vi "SetList.vi"() -> ()   [LabVIEW 2013]
uses:
  ColumnVIs/Column/Column.lvclass
  ColumnVIs/ModeCol/ModeCol.lvclass
  ColumnVIs/GroupCol/GroupCol.lvclass
  ColumnVIs/DigitalCol/DigitalCol.lvclass
  ColumnVIs/TriggerCol/TriggerCol.lvclass
  ColumnVIs/SingleValCol/SingleValCol.lvclass
  <vilib>/event_ctls.llb/eventvkey.ctl
  <vilib>/Utility/miscctls.llb/LVRowAndColumnTypeDef.ctl
  TypeDefs/RowType.ctl
  TypeDefs/TableHistory.ctl
  TypeDefs/TableArray.ctl
  TypeDefs/AddDeviceRing.ctl
  DeviceVIs/Device/Device.lvclass
  TypeDefs/PreviousVersionSelect.ctl
  VariableManagerCodes/VariableManager/VariableManager.lvclass
  <vilib>/Utility/miscctls.llb/LVRowAndColumnUnsignedTypeDef.ctl
  PackedLibraries/LuaEvaluatorAPI.lvlibp/API/t_Caching_Expression_Evaluator_Methods_Table.ctl
  TypeDefs/ClickEvent.ctl
  <vilib>/Utility/miscctls.llb/LVPoint32TypeDef.ctl
  TypeDefs/SetListRefs.ctl
  <vilib>/Utility/error.llb/DialogType.ctl
  TypeDefs/SaveCluster.ctl
  <vilib>/Utility/miscctls.llb/LVStringsAndValuesArrayTypeDef_I32.ctl
  <vilib>/Utility/cursorutil.llb/Set Cursor (Icon Pict).vi
  VariableManagerCodes/API/VariableManagerAPI.lvlib
  Globals/UserFunctions.vi
  PackedLibraries/LuaEvaluatorAPI.lvlibp
panel:
  in  "Launch Viewer":bool
  out "Cycle Time (s)":dbl
  in  "UpdateHWI Button":bool
  in  "StopExperiment":bool
  in  "Run Seq Button":bool
  in  "Run Button":bool
  in  "Cycle":bool
  in  "RandomSequence":bool
  out "Procedure Name":string="test_branch"
  in  "Tab Control":T1(tab)=enum."Variables"
  in  "Resume Button":bool
  in  "Program only changes":bool=TRUE
  out "SequenceHistory":string[][](table)
  in  "File Number":i32
  in  "Program during MOT loading":bool
  in  "Additional wait time (s)":dbl
  out "Igor Inform String":string
  in  "FitCol2Text Button":bool
  in  "SetList Table":string[][](table)=[["initialize", "", "Ramp", "1", "1", "0", "0", "0", "0", "0", "0", "0", "0", "0", "0", "0", "0", "0", "0", "0", "0", "0", "0", "0", "0", "0", "0", "0", "0", "100m"]]
  in  "Undo":bool
  in  "Redo":bool
  in  "Select Layout":i32(ring)=-1 items=["(On-the-fly)"=-2, "All"=-1]
  in  "ConfigLayoutsButton":bool
  in  "Add Device":T2 items=["Select Type...", "DDS", "Novatech", "NI Card", "Slave PB", "PTS via PB"]
  in  "ManageDevicesButton":bool
  in  "User defined functions":string="-- --------------------------------------------------------------------------\n-- RbYb Beatnote Command \"frequency\" functions\n--      These functions allow us to run a sequence using absolute frequency \n--      detuning by calculating the proper command \"frequency\"\n--\n--      NOTE: Only use one TA or Re \"comm\" function, or it isn't clear which setpoint will be used\n--\n--      18.Aug.2010: Updated Master AOM offset (40 --> 42.342).\n-----------------------------------------------------------------------------\nfunction TASlowComm(Detuning,AOM)\n    return (-1*Detuning+1126.48-60.32-42.342-2*AOM)/8\n   --positive detuning is BLUE detuned, zero detuning sets TA slower beam to the 87-Rb F=2 to F'=3\nend\n\nfunction TAMOTComm(Detuning,AOM)\n    return (-1*Detuning+1126.48-60.32-42.342+AOM)/8\n   --positive detuning is BLUE detuned, zero detuning sets TA MOT beam to the 87-Rb F=2 to F'=3\nend\n\nfunction TAPComm(Detuning,AOM)\n    return (-1*Detuning+1126.48-60.32-42.342+AOM)/8\n   --positive detuning is BLUE detuned, zero detuning sets TA Probe beam to the 87-Rb F=2 to F'=3\nend\n\nfunction ReMOTComm(Detuning,AOM)\n    return (Detuning+6568.03-1126.48+60.32+42.342-2*AOM)/64\n    --positive detuning is BLUE detuned, zero detuning sets Repump MOT beam to the 87-Rb F=1 to F'=2\nend\n\nfunction ReSlowComm(Detuning,AOM)\n    return (Detuning+6568.03-1126.48+60.32+42.342+2*AOM)/64\n    --positive detuning is BLUE detuned, zero detuning sets Repump slower beam to the 87-Rb F=1 to F'=2\nend\n\n--RbLi Probe (transverse coolign launch)\nfunction PComm(Detuning)\n    return (-1*Detuning+986.16)/8\n    --positive detuning is BLUE detuned, zero detuning sets Repump slower beam to the 87-Rb F=1 to F'=2\nend\n\n-- Creates an exponential ramp from A to B in tEnd seconds\n-- useful for stopping a ramp at different times to measure T, N\nfunction ExpRampStep(t, a, b, tau, tEnd)\n   return (b - a*exp(tEnd / tau) + (a-b)*exp(t/tau))/ ( 1 - exp(tEnd / tau) );\nend\n\nfunction ExpRampEnd(tEv, a, b, tau, tEnd)\n   return (b - a*exp(tEnd / tau) + (a-b)*exp(tEv/tau))/ ( 1 - exp(tEnd / tau) );\nend\n\nfunction ExpRamp2(t,a,tau)\n   return a*exp(-t/tau)\nend\n\nfunction ExpRamp2End(tEnd,a,tau)\n   return a*exp(-tEnd/tau)\nend\n\n-- Added log chip amplifier (1 V per decade) so now we provide linear ramp to get exponential\n--     note: log() is base 'e', log10 base '10'\nfunction LineEvap(t,a,tau)\n   return 1.027*(log10(a)-t/(2.30*tau))+0.0343\nend\n\n-- final value log(V) for LineEvap\nfunction LineEvapEnd(tEnd,a,tau)\n   return 1.027*(log10(a)-tEnd/(2.30*tau))+0.0343\nend\n\n-- Convert real dipole power to log chip request V\nfunction PtoV(pow)\n   return 1.010*log10(pow/0.770)\nend\n\n-- Convert 532 horizontal (main) beam power (in mW) to V-req\nfunction PtoV532m(pow)\n   return 1.01378*log10(pow/0.54672)\nend\n\n-- Convert 532 vertical (crossing) beam power (in mW) to V-req\nfunction PtoV532c(pow)\n   return 1.03459*log10(pow/0.619665)\nend\n\n-- Convert 1064 horizontal (main) beam power (in mW) to V-req\nfunction PtoV1064m(pow)\n   return 1.0035*log10(pow/1.2104)\nend\n----------------------------------------\n-- The following functions are part of the \"standard load\" of functions and should not be messed with\n-- They are here for reference only.\n-- Please add any user functions above this comment\n-- -------------------------------------------------------------------------------------------\n\n-- Creates a linear ramp from A to B\nfunction LineRamp(f, Initial, Final)\n    return (1-f)*Initial + f*Final;\nend\n\n-- Creates an exponential ramp from A to B\nfunction ExpRamp(t, a, b, tau)\n   return (b - a*exp(tMax / tau) + (a-b)*exp(t/tau))/ ( 1 - exp(tMax / tau) );\nend\n\n-- Creates a sinewave\nfunction SinRamp(t,Offset,A,Freq, Phase)\n    return Offset + A * sin(2*pi*Freq*t + Phase)\nend\n\n-- Creates a blackman pulse\nfunction Blackman(f, Offset, A)\n    return Offset +  A*sqrt(0.5*cos(3.1415*(2*f-1))+0.08*cos(2*pi*(2*f-1))+0.42);\nend\n\n-- Creates a half-gauss ramp\nfunction HalfGaussRamp(t, a, b, Width)\n    local y;\n    y = exp(-(tMax^2)/Width^2);\n    y = (a -  b*y)/(1-y)  +  ((b-a)/(1-y))*exp(-((t-tMax)^2)/Width^2);\n    return y;\nend\n\n-- Creates an \"O'Hara\" ramp from A to B, for dipole evaporation\nfunction EvapRamp(t, a, b, tau)\n   local y;\n  y = log(a/b) / log(1+tMax/tau);\n  y = a * (1+t/tau)^(-y);\n  return y;\nend\n"
  out "Loading Text":string="Loading..."
  in  "Version Selection":T3=enum."Load DDS 4.10"
  in  "Old HWGlobals Path":path=path "C:/Experiment/Data Acquisition/Hardware Control/Hardware/2014/6Jun2014_PowerCal" caption="This file has not been loaded or saved"
  in  "Old HWGlobals History":string(combo)
  in  "Old Procedure Path":path=path "C:/Experiment/Data Acquisition/Hardware Control/procedures/Benchmarks/12Feb2014_RbQuad" caption="This file has not been loaded or saved"
  in  "Old Procedure History":string(combo)
  in  "Load Old":bool
  in  "Load Recent":string(combo)
  in  "Save to Disk":bool
  in  "Load from Disk":bool
  out "Loaded Version":string="testing"
  out "Table error":errorcluster
  out "Run/Sequence Error":errorcluster
  out "Update Error":errorcluster
  out "Index Values":T4
  out "#chg":i16
  out "Defer Pnl Upd":bool=TRUE
  out "diag. loop cnt":i32
  out "Key Focus":bool
  out "Edit Position":T5={"Row"=-2, "Column"=-2}
  out "withinSelection?":bool
  out "Val Change":bool=TRUE
  out "Selection Size":T5
  out "Selection Start":T5={"Row"=25, "Column"=30}
  out "Char":i16
  out "VKey":T6
  out "withinData?":bool=TRUE
  out "data cols":i32=134
  out "data rows":i32=26
  out "Number of Rows":u32=36
  out "Number of Columns":u32=62
  in  "Devices":refnum<class "Device.lvclass">[](array[class])
  out "Devices queue":refnum<queue>
  out "DevNums":i32[](array[numeric])=[0, 0, 0, 0, 0, 0, 0, 0, 0, 0, 0, 0, 0, 0, 0, 0, 0, 0, 0, 0, 0, 0, 0, 0, 0, 0, 0, 0, 0, 0, 1, 1, 1, 1, 1, 1, 1, 1, 1, 1, 1, 1, 1, 1, 1, 1, 1, 1, 1, 1, 2, 2, 2, 2, 2, 2, 2, 2, 2, 2, 2, 2, 2, 2, 2, 2, 2, 2, 2, 2, 3, 3, 3, 3, 3, 3, 3, 3, 3, 3, 3, 3, 3, 3, 3, 3, 3, 3, 3, 3, 4, 4, 4, 4, 4, 4, 4, 4, 5, 5, 5, 5, 5, 5, 5, 5, 5, 5, 5, 5, 6, 6, 6, 6, 6, 6, 6, 6, 6, 6, 6, 6, 7, 7, 7, 7, 7, 7, 7, 7, 7, 7, 7, 7]
  out "Col array":refnum<class "Column.lvclass">[](array[class])
  out "Seq. Event":refnum<user-event>
  out "Update Event":refnum<user-event>
  out "Update Notifier":refnum<notifier>
  out "Dyn. Regist. Update Event":refnum<event-registration>
  out "Dyn.\nRegist.\nSeq.\nEvent":refnum<event-registration>
  out "Dyn.\nRegist.\nCycleX\nEvent":refnum<event-registration>
  out "CycleX Event":refnum<user-event>
  in  "row type":T7=enum."within data"
  out "Button\n(Mouse Down?)":u16
  in  "VariableManager":refnum<class "VariableManager.lvclass">=refnum
  out "Igor Inform Array":string[](array[string])
  out "Clipboard":string[][](array[string])
  out "Table History":T8
  in  "Diag. loop?":bool
  in  "PreserveHist?":bool
  out "Hist. size":i32=2
  in  "Defer Updates?":bool=TRUE
  in  "initialize?":bool
  in  "Debug: apply appearance":bool
  out "Viewer VI ref":refnum<vi>
  in  "quit":bool
  # "What do we actually need from old CycleX here?\n   - Inform Igor?\n   - Program changes/ during MOT load?"
  # "(not presently implemented)"
  # "Variable Manager will be initialized when the VI is run.\n\nIf it is currently running and you can see this message, then you've \"popped out\" the Variable manager.\nClose it with the \"red-x\" to replace it here."
  # "Note: For each index <idx>, the names <idx>_f and <idx>_max\nare also defined as the fractional sequence step and max steps."
  # "NOTE: these persist until LabVIEW is closed or you overwrite them."
  # "In the context of ramps several variables are passed or specified that may be used here:\n\n   - f the fractional position of a point in a ramp\n   - t the current time in a ramp\n   - dt the current timestep size.\n   - tMax the total duration of the ramp\n\ntemporary \"storage\":\n-- not functionality for strings (always treated as double)\nfunction bnot(a)\n   -- this \"(bool exp.) and b or c\" is equivalent to \"(bool exp.) ? b : c\" syntax.\n   -- caution: undefined variables evaluate to \"false\" so will NOT throw an error as argument\n   return a==0 and 1 or 0\nend"
  # "Present Version"
  # "Save/Load from present version (select single file):\nWe need to save the following:\n   - Devices (with the columns and data pushed from table first!)\n   - Layout ring (for layout names, #s)\n   - variables\n   - user functions\n   - ... ?"
  # "Load... and Save... bring up dialog box.\nLoad Recent will load the selected procedure. BUG: not a value change if select what's on top!"
  # "Previous Versions"
  # "Load from older versions (select Procedure and Hardware globals)\n(1) reformat old file to give device array\n(2) collect variables and send them to variable manager\n(3) load user functions\n(4) construct layouts, if any (at least a default \"all on\" layout)\n(5) ...?"
  # "Most of these controls/indicators MUST exist. At the bottom and right are some diagnostics."
  # "\"Diagnostics\" we can't delete:\nRow Type, ..."
  # "(must abort to stop,\nstill better to QUIT first)"
  # "diagnostics:"
  # "presently not set\nfor row header"
  # "The table size in (rows, cols) is NOT same as\nthe size of the data array displayed in table."
  # "SetList was developed for the JQI neutral atom cooling/traping groups. \nPrimary contributions authored by Zack Seigel, Creston Herold, Joe Tiamsuphat, Bob Wyllie, Zach Smith.\n\nFAQs\n------\n * How are digital variables interpreted?\n     Any value not equal to 0 is high, only 0 is low.\n\n * What does Ramp mean?\n     Slave devices will be triggered (if necessary) during a Ramp line with a period given by \"Step.\" The output\n     is determined with Lua \"User Functions\" and the reserved f,t variables described on that tab.\n     Master (PulseBlaster) channels will output a *static* output during ramps. That means functions of f or t\n     will only be evaluated at their *first* point for Master channels.\n\n * How do you use Loop - EndLoop?\n     The \"Step\" column on a Loop line is for # loops and is ignored on an EndLoop line. Nesting is supported\n     up to 7 levels deep, but only Master (PulseBlaster) outputs can change. Therefore Ramps are not allowed \n     within loops.\n\n * How does Halt work?\n     On a Halt line, the Master (PulseBlaster) will change to the selected outputs and then wait for a trigger.\n     Upon receiving a trigger (hardware or software), it will wait for the specified Delay and then go to the \n     next instruction.\n\n * Where can I learn more?\n     Complete documentation of this code, including adding your own custom device can be found on the\n     JQI wiki (https://jqi-wiki.physics.umd.edu, login required)."
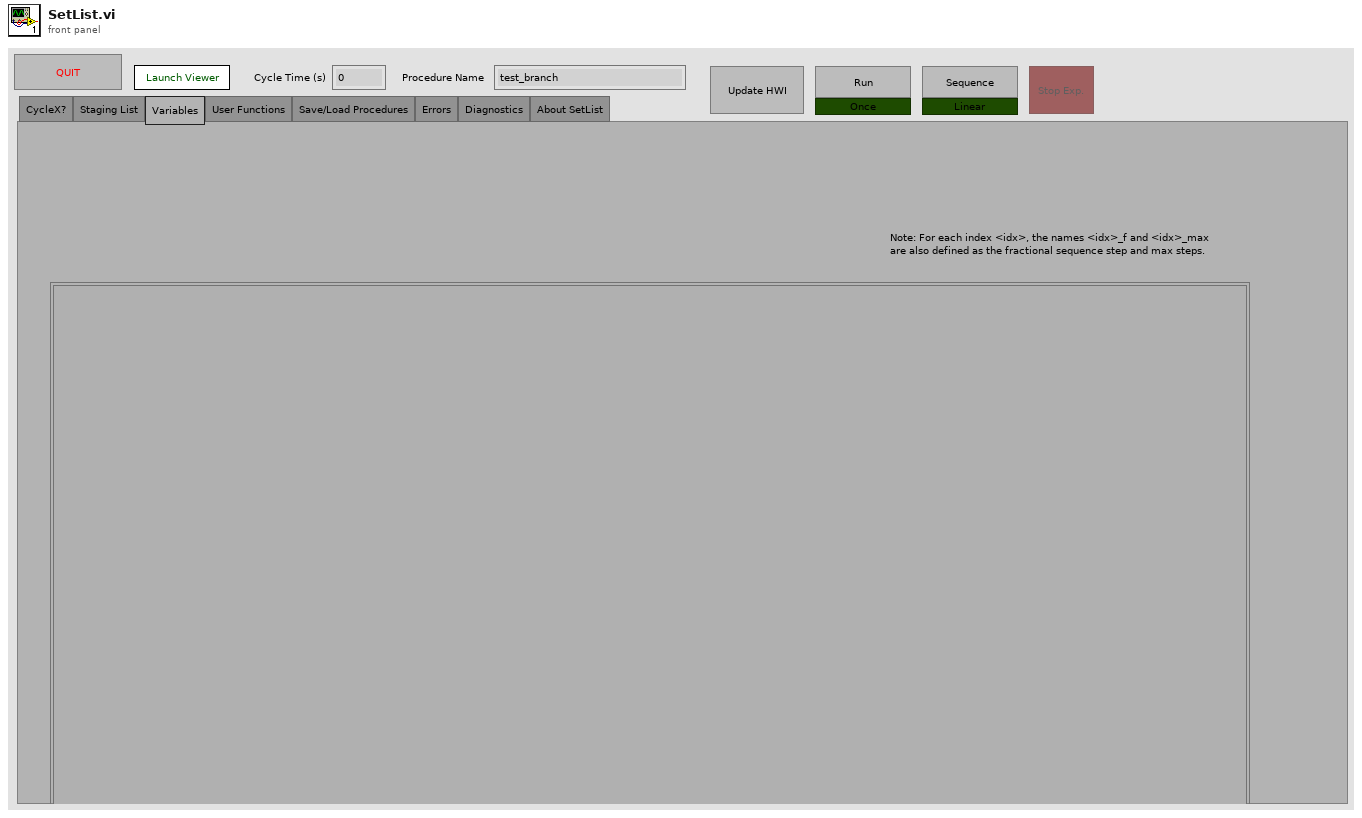
[diagram p1: front panel]
types:
  T1 = enum32{"CycleX?", "Staging List", "Variables", "User Functions", "Save/Load Procedures", "Errors", "Diagnostics", "About SetList"}
  T2 = typedef "AddDeviceRing.ctl" = u16
  T3 = typedef "PreviousVersionSelect.ctl" = enum32{"Load PreDDS 4.10", "Load early 2009 files", "Load 2009-2010 files", "Load DDS 4.10", "Load v4.09"}
  T4 = typedef "LVRowAndColumnUnsignedTypeDef.ctl" = cluster{"Row":u32, "Column":u32}
  T5 = typedef "LVRowAndColumnTypeDef.ctl" = cluster{"Row":i32, "Column":i32}
  T6 = typedef "eventvkey.ctl" = enum16{"ASCII", "Enter", "Return", "Shift", "Ctrl", "Alt", "Cmd", "Opt", "Caps", "NumLock", "Clear", "Break", "Up", "Down", "Left", "Right", "Insert", "Delete", "Home", "End", "PageUp", "PageDown", "Escape", "Help", "Pause", "ScrollLock", "F1", "F2", "F3", "F4", "F5", "F6", "F7", "F8", "F9", "F10", "F11", "F12", "F13", "F14", "F15", "F16", "F17", "F18", "F19", "F20", "F21", "F22", "F23", "F24", "Play", "VolumeUp", "VolumeDown", "Mute", "Two Byte Char"}
  T7 = typedef "RowType.ctl" = enum16{"below data", "within data", "column header", "first row"}
  T8 = typedef "TableHistory.ctl" = cluster{"OldTable Array":T9, "Undo pointer":i32}
  T9 = typedef "TableArray.ctl" = cluster{"OldTable":string[][]}[]
  T10 = typedef "LuaEvaluatorAPI.lvlibp/t_Caching_Expression_Evaluator_Methods_Table.ctl" = enum16{"set", "get", "eval", "assign", "isvalid", "execute", "evaltable", "close"}
  T11 = enum8{"Enabled", "Disabled", "Disabled and Grayed Out"}
  T12 = typedef "ClickEvent.ctl" = cluster{"CtlRef":refnum<vi>, "Coords":T13, "Button":u16, "Mods":cluster{"Double Click":bool, "Menu Key":bool}, "PlatMods":cluster{"Shift":bool, "Ctrl":bool, "Alt":bool, "Cmd":bool, "Opt":bool}}
  T13 = typedef "LVPoint32TypeDef.ctl" = cluster{"Horizontal":i32, "Vertical":i32}
  T14 = typedef "SetListRefs.ctl" = cluster{"Clipboard":refnum<vi>, "Layout Ring Refnum":refnum<vi>, "Col Array Ref in":refnum<vi>, "VariableManagerRef":refnum<vi>, "Table CtlRef In":refnum<vi>, "Table History ref":refnum<vi>, "Devices queue":refnum<queue>}
  T15 = typedef "SaveCluster.ctl" = cluster{"Version":string, "Devices":refnum<class "Device.lvclass">[], "Select Layout":i32, "Layout:Strings And Values []":T16, "User defined functions":string, "VariableManager":refnum<class "VariableManager.lvclass">}
  T16 = typedef "LVStringsAndValuesArrayTypeDef_I32.ctl" = cluster{"String":string, "Value":i32}[]
  T17 = cluster{"Shift":bool, "Ctrl":bool, "Alt":bool, "Cmd":bool, "Opt":bool}
  T18 = typedef "ClickReturn.ctl" = cluster{"Button":u16, "Mods":cluster{"Double Click":bool, "Menu Key":bool}, "PlatMods":cluster{"Shift":bool, "Ctrl":bool, "Alt":bool, "Cmd":bool, "Opt":bool}, "Discard?":bool}
  T19 = typedef "DialogType.ctl" = u16
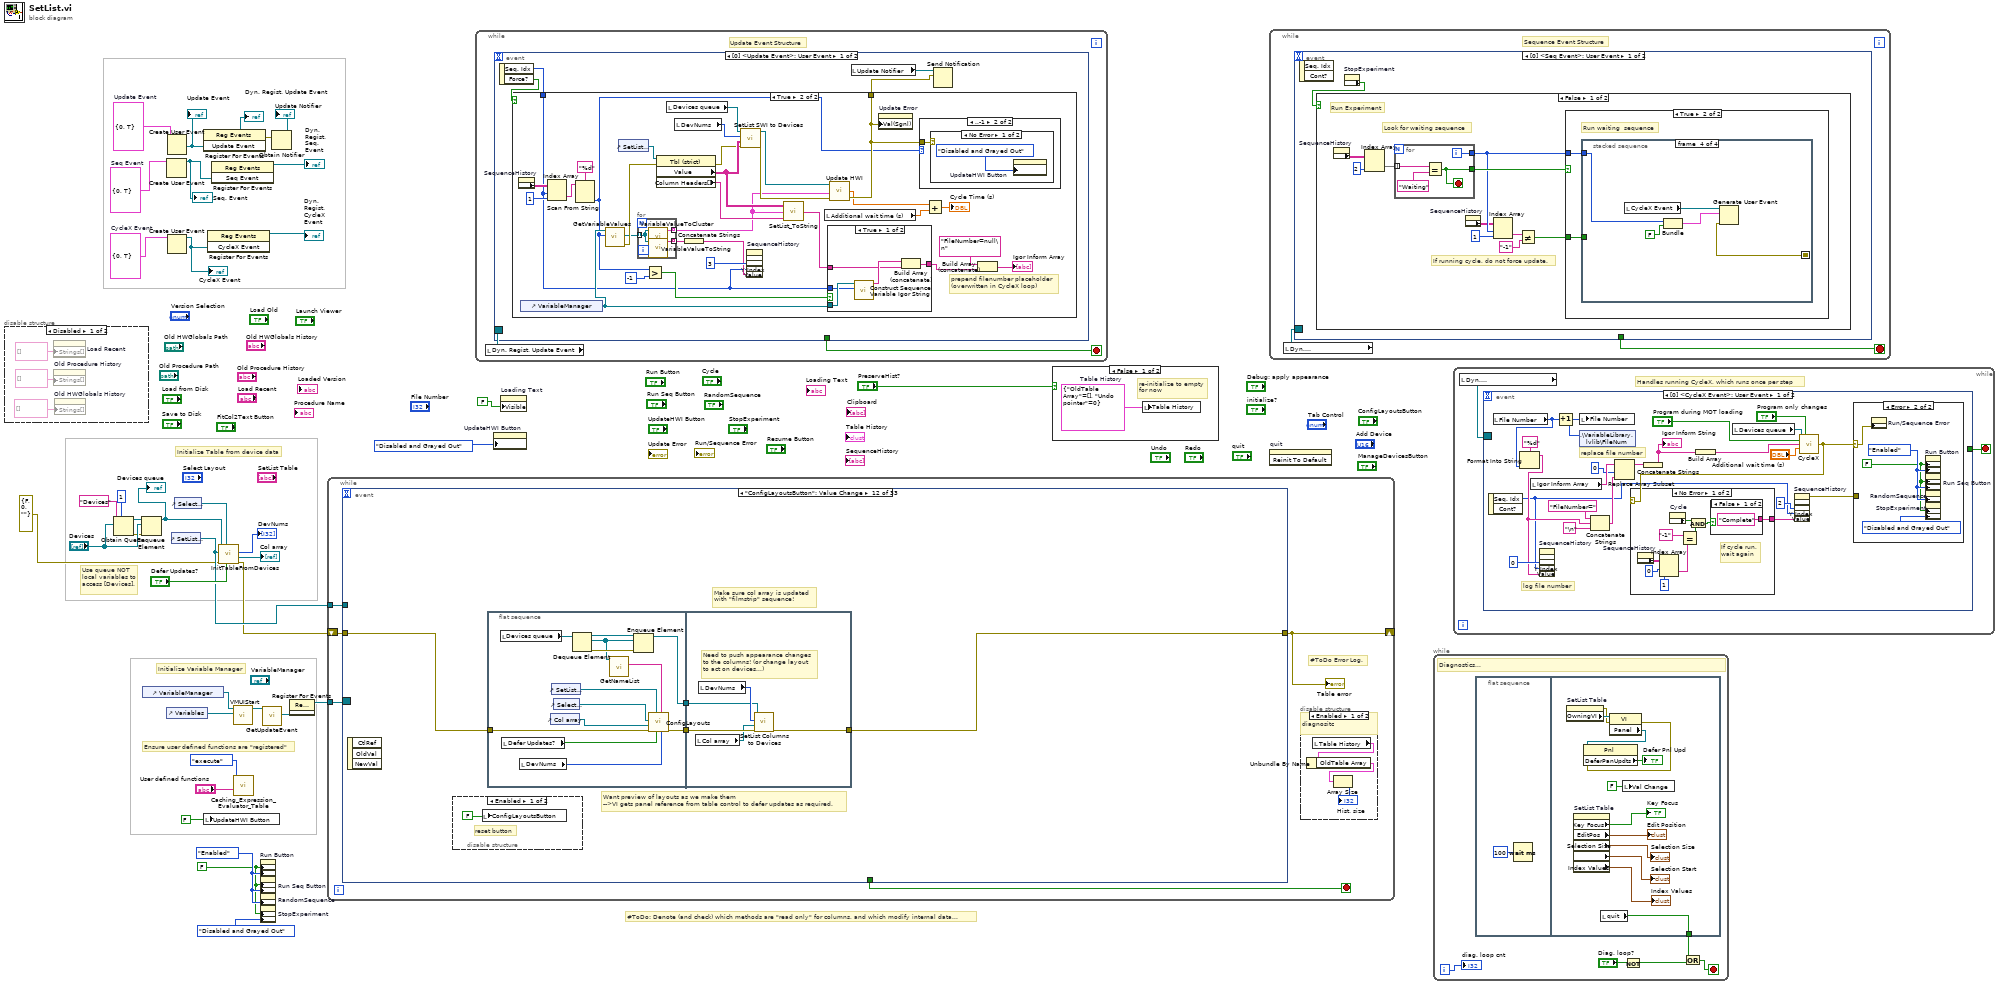
[diagram p0: block diagram]
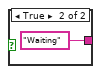
[diagram p2: hidden frame]
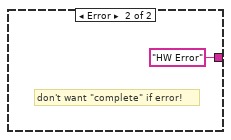
[diagram p3: hidden frame]
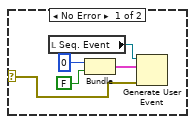
[diagram p4: hidden frame]
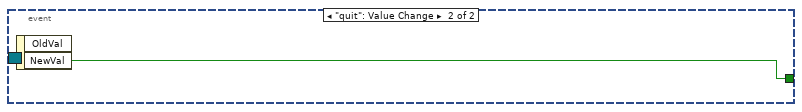
[diagram p5: hidden frame]
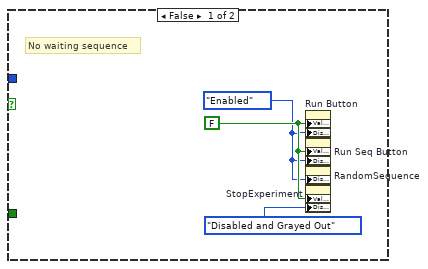
[diagram p7: hidden frame]
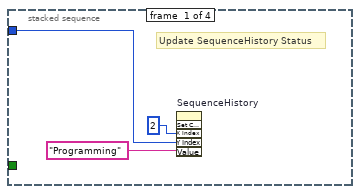
[diagram p8: hidden frame]
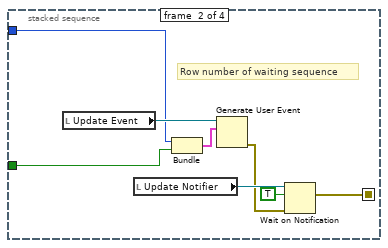
[diagram p9: hidden frame]
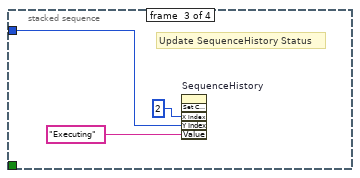
[diagram p10: hidden frame]
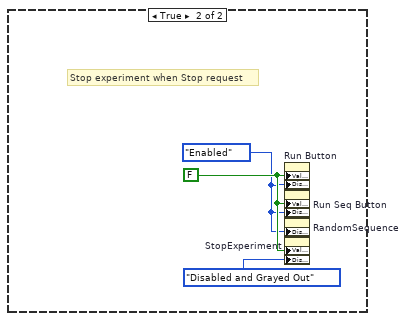
[diagram p11: hidden frame]
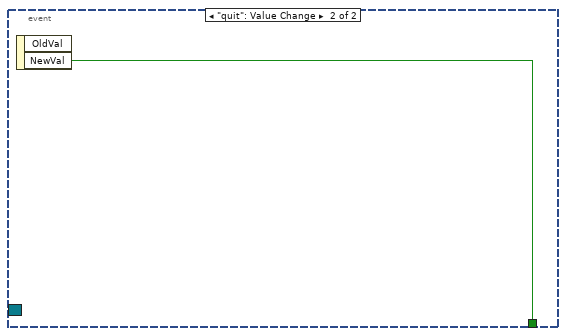
[diagram p12: hidden frame]
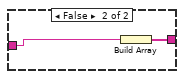
[diagram p16: hidden frame]
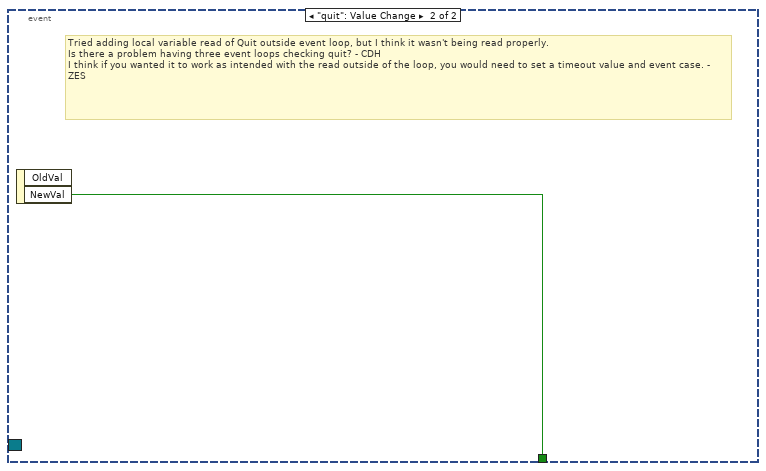
[diagram p17: hidden frame]
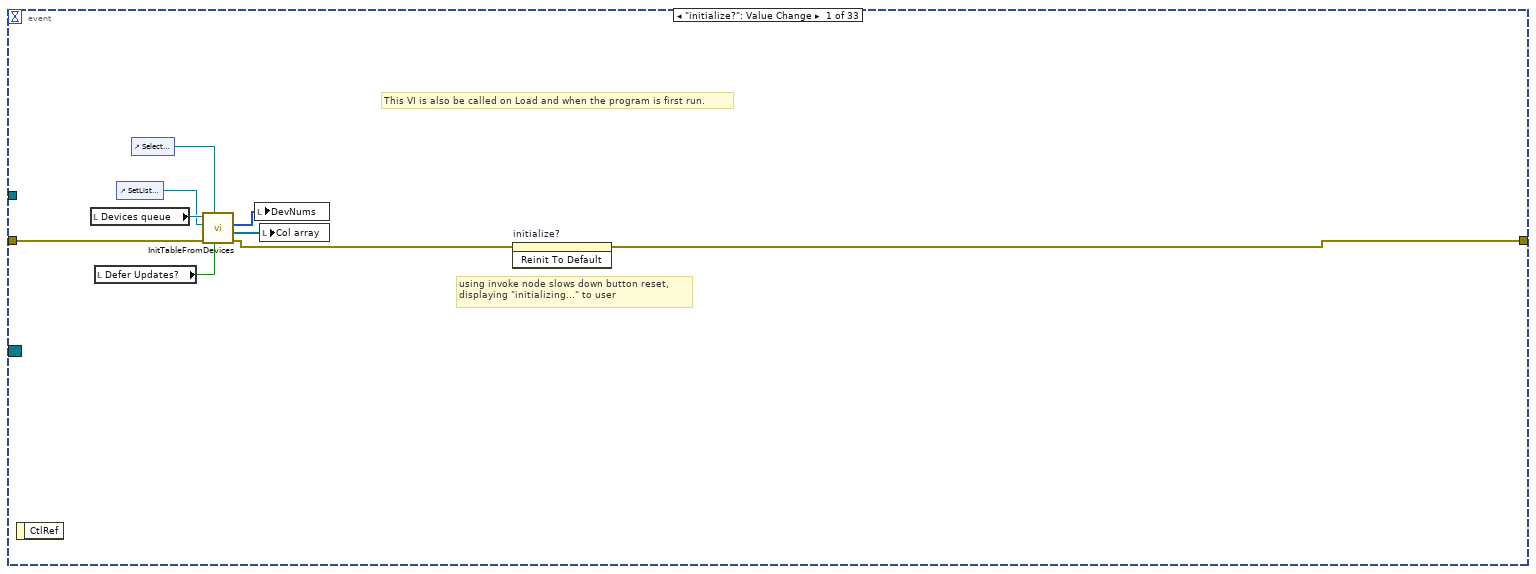
[diagram p20: hidden frame]
diagram:
  w14 = T11."Enabled" ("Disabled")
  w13 = FALSE
  w25 = cluster{"Seq. Idx":i32, "Cont?":bool} {"Seq. Idx"=0, "Cont?"=TRUE}  # CycleX Event
  w35 = cluster{"Seq. Idx":i32, "Cont?":bool} {"Seq. Idx"=0, "Cont?"=TRUE}  # Seq Event
  w36 = cluster{"Seq. Idx":i32, "Force?":bool} {"Seq. Idx"=0, "Force?"=TRUE}  # Update Event
  # "Use queue NOT\nlocal variables to\naccess [Devices]."
  # "Ensure user defined functions are \"registered\""
  # "Initialize Variable Manager"
  # "Initialize Table from device data"
  # "#ToDo: Denote (and check) which methods are \"read only\" for columns, and which modify internal data..."
  n1 = disable-structure shown="Disabled" {
    frame Disabled {
      n2 = property on="Load Recent" class="CmbBox"("Strings[]"=string[] [] ("Strings []")) -> ()  [unwired: 2 in, 2 out]
      n3 = property on="Old Procedure History" class="CmbBox"("Strings[]"=string[] [] ("Strings []")) -> ()  [unwired: 2 in, 2 out]
      n4 = property on="Old HWGlobals History" class="CmbBox"("Strings[]"=string[] [] ("Strings []")) -> ()  [unwired: 2 in, 2 out]
    }
    frame Enabled {
    }
  }
  n5 = Obtain Queue(max queue size (-1, unlimited)=1, name (unnamed)="Devices", element data type="Devices") -> (queue out=w6:refnum<queue>, error out=w5:errorcluster)  [unwired: 2 in, 1 out]
  n6 = Enqueue Element(queue=w6, element="Devices", error in (no error)=w5) -> (queue out=w4:refnum<queue>)  [unwired: 1 in, 2 out]
  "Devices queue" <- w4
  n7 = control-ref of="VariableManager"() -> (w17:refnum<vi>)
  n8 = control-ref of="Variables"() -> (w16:refnum<vi>)
  n9 = Create User Event(user event datatype=w35) -> (user event=w22:refnum<user-event>)  [unwired: 1 in, 1 out]
  "Seq. Event" <- w22
  n10 = Create User Event(user event datatype=w36) -> (user event=w37:refnum<user-event>)  [unwired: 1 in, 1 out]
  "Update Event" <- w37
  n11 = Create User Event(user event datatype=w25) -> (user event=w24:refnum<user-event>)  [unwired: 1 in, 1 out]
  "CycleX Event" <- w24
  n12 = control-ref of="SetList Table"() -> (w19:refnum<vi>)
  n13 = control-ref of="Select Layout"() -> (w31:refnum<vi>)
  n14 = register-events(w37) -> (reference out=→"Dyn. Regist. Update Event":refnum<event-registration>, error out=w33:errorcluster)  [unwired: 2 in]
  n15 = local write "UpdateHWI Button"(FALSE ("UpdateHWI Button")) -> ()
  n16 = register-events(w24) -> (reference out=→"Dyn.\nRegist.\nCycleX\nEvent":refnum<event-registration>)  [unwired: 2 in, 1 out]
  n17 = register-events(w22) -> (reference out=→"Dyn.\nRegist.\nSeq.\nEvent":refnum<event-registration>)  [unwired: 2 in, 1 out]
  n18 = call "InitTableFromDevices.vi"("Defer Updates? (T)"="Defer Updates?", "Layout Ref"=w31, "error in (no error)"=errorcluster {"status"=FALSE, "code"=0, "source"=""} ("error out"), "Table Ref in"=w19, "Devices queue"=w4) -> ("error out"=w18:errorcluster, "Col array"=→"Col array":refnum<class "Column.lvclass">[], "DevNums"=→"DevNums":i32[])  [unwired: 3 in, 1 out]
  n19 = call "VMUIStart.vi"("SubPanelRef"=w16, "VariableManagerRef in"=w17) -> ("VariableManagerRef out"=w12:refnum<vi>)  [unwired: 8 in, 1 out]
  n20 = call "Caching_Expression_Evaluator_Table.vi"("method"=t_Caching_Expression_Evaluator_Methods_Table."execute", "expression/scriptlet"="User defined functions") -> ()  [unwired: 11 in, 3 out]
  n21 = property on="Run Button" class="Bool (strict)"("Value"=w13, "DisabledEnum"=w14) -> ()  [unwired: 2 in, 2 out]
  n22 = property on="Run Seq Button" class="Bool (strict)"("Value"=w13, "DisabledEnum"=w14) -> ()  [unwired: 2 in, 2 out]
  n23 = property on="RandomSequence" class="Bool (strict)"("DisabledEnum"=w14) -> ()  [unwired: 2 in, 2 out]
  n24 = property on="StopExperiment" class="Bool (strict)"("Value"=w13, "DisabledEnum"=T11."Disabled and Grayed Out" ("Disabled")) -> ()  [unwired: 2 in, 2 out]
  n25 = call "GetUpdateEvent.vi"("VariableManagerRef in"=w12) -> ("UpdateEvent"=w11:refnum<user-event>)  [unwired: 8 in, 2 out]
  n26 = Obtain Notifier(notification data type=w33) -> (notifier out=→"Update Notifier":refnum<notifier>)  [unwired: 3 in, 2 out]
  n27 = register-events(w11) -> (reference out=w10:refnum<event-registration>)  [unwired: 2 in, 1 out]
  n28 = while {
    shift-right: [w44] -> _
    shift-left: w18 -> [w45]
    tunnel: w19 -> [w43]
    tunnel: w10 -> [w42]
    stop <- w46 stop-if-true
    # "#ToDo Error Log."
    n29 = event shown="[11] \"ConfigLayoutsButton\": Value Change" {
      selector: w42 -> [_ _ _ _ _ _ _ _ _ _ _ _ _ _ _ _ _ _ _ _ _ _ _ _ _ _ _ _ _ _ _ _ _]
      dyn-events: _ -> [_ _ _ _ _ _ _ _ _ _ _ _ _ _ _ _ _ _ _ _ _ _ _ _ _ _ _ _ _ _ _ _ _]
      timeout: _ -> [_ _ _ _ _ _ _ _ _ _ _ _ _ _ _ _ _ _ _ _ _ _ _ _ _ _ _ _ _ _ _ _ _]
      tunnel: [_ _ _ _ _ _ _ _ _ _ _ _ _ _ _ w404 _ _ _ _ _ _ _ _ _ _ _ _ _ _ _ _ _] -> w46
      tunnel: [w50 w60 w114 w214 _ w249 w274 w284 w287 w296 w312 w318 w340 w359 _ w391 w413 w439 _ _ _ _ _ _ _ w583 _ _ w596 _ _ _ _] -> w44
      tunnel: w45 -> [w53 w64 w113 w215 w225 w248 w282 w285 w288 w292 w313 w320 w345 w356 _ w398 w412 w441 _ _ _ _ _ _ _ w579 _ _ _ _ _ _ _]
      tunnel: w43 -> [_ _ _ _ _ _ _ _ _ _ w311 _ w344 w354 _ _ w410 w436 _ _ _ _ _ _ _ _ _ _ _ _ _ _ _]
      event "initialize?": Value Change {
        # "using invoke node slows down button reset,\ndisplaying \"initializing...\" to user"
        # "This VI is also be called on Load and when the program is first run."
        n30 = event-data() -> ()  [unwired: 1 in, 1 out]
        n31 = local read "Devices queue"() -> (w58:refnum<queue>)
        n32 = local read "Defer Updates?"() -> (w52:bool)
        n33 = control-ref of="SetList Table"() -> (w55:refnum<vi>)
        n34 = control-ref of="Select Layout"() -> (w54:refnum<vi>)
        n35 = call "InitTableFromDevices.vi"("Defer Updates? (T)"=w52, "Layout Ref"=w54, "error in (no error)"=w53, "Table Ref in"=w55, "Devices queue"=w58) -> ("error out"=w51:errorcluster, "Col array"=w56:refnum<class "Column.lvclass">[], "DevNums"=w57:i32[])  [unwired: 3 in, 1 out]
        n36 = local write "DevNums"(w57) -> ()
        n37 = local write "Col array"(w56) -> ()
        n38 = invoke on="initialize?" class="Bool (strict)" method="Reinit To Default"(error in=w51) -> (error out=w50:errorcluster)  [unwired: 2 in, 2 out]
      }
      event "SetList Table": Value Change {
        # "presently assumes value change to single cell!"
        # "need to catch digital value change ->appear change"
        # "Value change (e.g. tab and enter) shouldn't change array size.\nOnly way to add/remove rows is through mouse clicks..."
        # "monitor sizes"
        n39 = event-data() -> ("CtlRef"=w63:refnum<vi>, "OldVal"=w65:string[][], "NewVal"=w62:string[][])  [unwired: 1 in]
        n40 = property on="Property Node" class="Tbl (strict)"(reference=w63, error in=w64) -> (error out=w61:errorcluster, "Number of Rows"=→"Number of Rows":u32, "Number of Columns"=→"Number of Columns":u32)  [unwired: 1 out]
        n41 = Array Size(array=w65) -> (size(s)=w73:i32[])
        n42 = Array Size(array=w62) -> (size(s)=w76:i32[])
        n43 = Index Array(array=w76) -> (element #1=w72:i32, element #2=w71:i32)  [unwired: 2 in]
        n44 = Index Array(array=w73) -> (element #1=w68:i32, element #2=w67:i32)  [unwired: 2 in]
        "data rows" <- w68
        "data cols" <- w67
        n45 = Equal?(x=w72, y=w68) -> (x = y?=w69:bool)
        n46 = Equal?(x=w71, y=w67) -> (x = y?=w70:bool)
        n47 = And(x=w69, y=w70) -> (x .and. y?=w66:bool)
        n48 = case shown="False" w66 {
          tunnel: w65 -> [w78 w84]
          tunnel: w62 -> [_ w88]
          tunnel: w61 -> [w77 w85]
          tunnel: [w77 w89] -> w60
          frame False {
            # "non-allowed resize:\nrevert back to previous table"
            # "Changed outside existing data; discard"
            n49 = local write "SetList Table"(w78) -> ()
          }
          frame True {
            # "Change within existing data"
            n50 = Not Equal?(x=w84, y=w88) -> (x != y?=w82:bool[][])
            n51 = Boolean To (0,1)(Boolean=w82) -> (0, 1=w81:i16[][])
            n52 = Add Array Elements(numeric array=w81) -> (sum=→"#chg":i16)
            n53 = Or Array Elements(Boolean array=w82) -> (logical OR=w87:bool)
            n54 = control-ref of="Table History"() -> (w83:refnum<vi>)
            n55 = call "SaveToTblHist.vi"("error in (no error)"=w85, "OldTable (reset)"=w84, "Table History ref"=w83) -> ("error out"=w86:errorcluster)  [unwired: 8 in]
            n56 = case shown="True" w87 {
              tunnel: w82 -> [_ w103]
              tunnel: w86 -> [w90 w91]
              tunnel: [w90 w99] -> w89
              tunnel: w88 -> [_ w95]
              frame False {
                # "No value change! (debugging event)"
              }
              frame True {
                # "new val"
                # "Find col, row of value change; notify column"
                n57 = for {
                  tunnel: w103 -> [w107] mode=indexing
                  tunnel: [w107] -> w102
                  tunnel: [w106] -> w94
                  i -> [w106]
                  stop <- w108 stop-if-true
                  # "which row?"
                  n58 = Or Array Elements(Boolean array=w107) -> (logical OR=w108:bool)
                }
                n59 = for {
                  tunnel: w102 -> [w104] mode=indexing
                  tunnel: [w105] -> w93
                  i -> [w105]
                  stop <- w104 stop-if-true
                  # "which col?"
                }
                n60 = Bundle By Name(cluster=T5 {"Row"=0, "Column"=0} ("Cell Position"), "Row"=w94, "Column"=w93) -> (w97:T5)
                n61 = Index Array(array=w95, index (row)=w94, index (col)=w93) -> (element=w92:string)
                n62 = local read "Col array"() -> (w100:refnum<class "Column.lvclass">[])
                n63 = Index Array(array=w100, index=w93) -> (element=w96:refnum<class "Column.lvclass">)
                n64 = control-ref of="SetList Table"() -> (w98:refnum<vi>)
                n65 = call-dynamic "ValChange.vi"("Value"=w92, "error in (no error)"=w91, "Table CtlRef In"=w98, "Cell Position"=w97, "Column in"=w96) -> ("error out"=w99:errorcluster)  [unwired: 4 in, 2 out]
              }
            }
            n66 = property on="UpdateHWI Button" class="Bool (strict)"("DisabledEnum"=T11."Enabled" ("Disabled")) -> ()  [unwired: 2 in, 2 out]
          }
        }
        "Val Change" <- TRUE ("Val Change")
      }
      event "SetList Table": Key Down? {
        # "#ToDo: Copy/Paste not working... \nAccording to the LabVIEW help files, Ctrl-V or any menu-shortcut CANNOT be repurposed,\neven if the menus are hidden!"
        # "Selection start is initially placed at the edit on mouse press, so it provides (row, col). However keyboard motion (default Return, Tab behavior) doesn't move it.\nTo re-enable keyboard navigation (and to add arrow keys), one needs to force selection start to move so it can be checked on each key stroke!\n\nRevisit this: After mouse handling \"paradigm\" has been re-worked, this should be easier to include. See Sandbox/TableSanbox.vi (Key Down event) for ideas."
        n67 = event-data() -> ("CtlRef"=w117:refnum<vi>, "Char"=w121:i16, "VKey"=w120:T6, "PlatMods"=w119:T17)  [unwired: 1 in, 3 out]
        "VKey" <- w120
        "Char" <- w121
        n68 = local read "Devices queue"() -> (w109:refnum<queue>)
        n69 = control-ref of="Table History"() -> (w111:refnum<vi>)
        n70 = control-ref of="Col array"() -> (w115:refnum<vi>)
        n71 = control-ref of="Select Layout"() -> (w112:refnum<vi>)
        n72 = Unbundle By Name(w119) -> ("Ctrl"=w118:bool)
        n73 = call "ModeFromDevices.vi"("Devices queue"=w109) -> ("Mode Col"=w110:i32)  [unwired: 9 in, 1 out]
        n74 = control-ref of="Clipboard"() -> (w116:refnum<vi>)
        n75 = case shown="118" w121 {
          tunnel: [w124 w127 eventvkey."Enter" ("VKey") w137 w169] -> w122
          tunnel: w120 -> [w124 w126 _ w136 w168]
          tunnel: w118 -> [_ _ _ w138 w170]
          tunnel: w117 -> [_ _ _ w135 w167]
          tunnel: w113 -> [w123 w125 w130 w134 w166]
          tunnel: w116 -> [_ _ _ w133 w165]
          tunnel: w115 -> [_ _ _ _ w164]
          tunnel: [w123 w125 w130 w132 w163] -> w114
          tunnel: w112 -> [_ _ _ _ w162]
          tunnel: w110 -> [_ _ _ _ w161]
          tunnel: w111 -> [_ _ _ _ w160]
          frame Default {
          }
          frame 0 {
            # "Choose how to handle \"navigation\" keys.\nchar0: arrow keys, enter, return, Shift, Caps, Insert, Ctrl, F-keys"
            n76 = case shown="\"Return\"" w126 {
              selector: w126 -> [w128 _]
              tunnel: [w128 eventvkey."Enter" ("VKey")] -> w127
              frame Default {
              }
              frame "Return" {
                # "Enter (char 0) = num pad key, accept value (remove key focus)\nReturn (char 0) = keyboard enter, edit next."
              }
            }
          }
          frame 9 {
            # "Tab, shift+Tab (char 9) = move edit to right, left.\nSet to Enter to discard \"edit movement\":"
          }
          frame 99 {
            # "c = ASCII char 99: Copy selected cells to clipboard if selection exists."
            n77 = case shown="False" w138 {
              tunnel: [w140 w143] -> w137
              tunnel: w136 -> [w140 w142]
              tunnel: w135 -> [_ w152]
              tunnel: w134 -> [w139 w151]
              tunnel: w133 -> [_ w144]
              tunnel: [w139 w141] -> w132
              frame False {
                # "CTRL not pressed (pass along c-press!)"
              }
              frame True {
                # "non-zero selection?"
                # "user pressed CTRL-C"
                n78 = property class="Tbl (strict)"(reference=w152, error in=w151) -> (reference out=w145:refnum<vi>, error out=w146:errorcluster, "Selection Size"=w149:T5)
                n79 = Greater Than 0?(x=w149) -> (x > 0?=w148:cluster{"Row":bool, "Column":bool})
                n80 = Cluster To Array(cluster=w148) -> (array=w150:bool[])
                n81 = And Array Elements(Boolean array=w150) -> (logical AND=w147:bool)
                n82 = case shown="True" w147 {
                  tunnel: w146 -> [w153 w159]
                  tunnel: w145 -> [_ w158]
                  tunnel: w144 -> [_ w157]
                  tunnel: [w154 w156] -> w143
                  tunnel: w142 -> [w154 w156]
                  tunnel: [w153 w155] -> w141
                  frame False {
                    # "no selection present"
                  }
                  frame True {
                    # "copy selection"
                    n83 = call "CopySelectedCells.vi"("Clipboard"=w157, "error in (no error)"=w159, "Table CtlRef In"=w158) -> ("error out"=w155:errorcluster)  [unwired: 7 in, 1 out]
                  }
                }
              }
            }
          }
          frame 118 {
            # "v = ASCII char 118: Copy selected cells to clipboard if selection exists."
            n84 = case shown="False" w170 {
              tunnel: [w172 w180] -> w169
              tunnel: w168 -> [w172 w179]
              tunnel: w167 -> [_ w189]
              tunnel: w166 -> [w171 w188]
              tunnel: w165 -> [_ w181]
              tunnel: w164 -> [_ w178]
              tunnel: [w171 w176] -> w163
              tunnel: w162 -> [_ w175]
              tunnel: w161 -> [_ w174]
              tunnel: w160 -> [_ w173]
              frame False {
                # "CTRL not pressed (pass along c-press!)"
              }
              frame True {
                # "non-zero selection?"
                # "user pressed CTRL-V"
                n85 = property class="Tbl (strict)"(reference=w189, error in=w188) -> (reference out=w182:refnum<vi>, error out=w183:errorcluster, "Selection Size"=w186:T5, "Selection Start"=w177:T5)
                n86 = Greater Than 0?(x=w186) -> (x > 0?=w185:cluster{"Row":bool, "Column":bool})
                n87 = Cluster To Array(cluster=w185) -> (array=w187:bool[])
                n88 = And Array Elements(Boolean array=w187) -> (logical AND=w184:bool)
                n89 = case shown="True" w184 {
                  tunnel: w183 -> [w190 w201]
                  tunnel: w182 -> [_ w200]
                  tunnel: w181 -> [_ w199]
                  tunnel: [w191 w198] -> w180
                  tunnel: w179 -> [w191 w198]
                  tunnel: w178 -> [_ w197]
                  tunnel: w177 -> [_ w196]
                  tunnel: [w190 w195] -> w176
                  tunnel: w175 -> [_ w194]
                  tunnel: w174 -> [_ w193]
                  tunnel: w173 -> [_ w192]
                  frame False {
                    # "no selection present"
                  }
                  frame True {
                    # "paste selection"
                    n90 = call "PasteSelectedCells.vi"("ModeCol Index"=w193, "Layout Ref"=w194, "Clipboard"=w199, "Table History ref"=w192, "error in (no error)"=w201, "Table CtlRef In"=w200, "Cell Start"=w196, "Col Array Ref in"=w197) -> ("error out"=w195:errorcluster)  [unwired: 1 in, 2 out]
                  }
                }
              }
            }
          }
        }
        n91 = event-data("VKey"=w122) -> ()  [unwired: 1 in, 1 out]
      }
      event "SetList Table": Mouse Down? {
        # "Note: need to check comments in shortcut menu events and update \"mouse down?\" references to new event."
        # "Filter Mouse Down click so that (1) columns can choose to change button (like mode column) and (2) so that some clicks can (sparingly!) be discarded.\nEach column will provide a MouseDown method.\n\nSortClicks (which ultimately called LeftClick) will be moved to Mouse Up event. (is this possible? if shortcut menu is activated, Mouse Up is skipped!)"
        # "No need for DeferPanUpdts here... In fact it screws up click-and-drag!"
        n92 = event-data() -> ("CtlRef"=w220:refnum<vi>, "Coords"=w219:T13, "Button"=w218:u16, "Mods"=w217:cluster{"Double Click":bool, "Menu Key":bool}, "PlatMods"=w216:T17)  [unwired: 1 in]
        "Button\n(Mouse Down?)" <- w218
        n93 = Bundle By Name(cluster=T12 {"CtlRef"=refnum, "Coords"={"Horizontal"=0, "Vertical"=0}, "Button"=0, "Mods"={"Double Click"=FALSE, "Menu Key"=FALSE}, "PlatMods"={"Shift"=FALSE, "Ctrl"=FALSE, "Alt"=FALSE, "Cmd"=FALSE, "Opt"=FALSE}} ("ClickEvent"), "CtlRef"=w220, "Coords"=w219, "Button"=w218, "Mods"=w217, "PlatMods"=w216) -> (w207:T12)
        n94 = local read "Col array"() -> (w212:refnum<class "Column.lvclass">[])
        n95 = control-ref of="Table History"() -> (w208:refnum<vi>)
        n96 = call "SortClicks.vi"("Table History ref"=w208, "error in (no error)"=w215, "ClickEvent in"=w207, "Col array in"=w212) -> ("error out"=w214:errorcluster, "Row Type"=w210:T7, "Click out"=w206:T18, "Col array out"=w211:refnum<class "Column.lvclass">[], "Update HWI?"=w209:bool, "withinData?"=→"withinData?":bool)  [unwired: 2 in]
        n97 = case shown="True" w209 {
          frame False {
          }
          frame True {
            n98 = property on="UpdateHWI Button" class="Bool (strict)"("DisabledEnum"=T11."Enabled" ("Disabled")) -> ()  [unwired: 2 in, 2 out]
          }
        }
        n99 = disable-structure shown="Disabled" {
          disable-tunnel: w211 -> [w222 _]
          frame Disabled {
            n100 = local write "Col array"(w222) -> ()
          }
          frame Enabled {
          }
        }
        n101 = local write "row type"(w210) -> ()
        n102 = Unbundle By Name(w206) -> ("Button"=w204:u16, "Mods"=w203:cluster{"Double Click":bool, "Menu Key":bool}, "PlatMods"=w202:T17, "Discard?"=w205:bool)
        n103 = event-data("Button"=w204, "Mods"=w203, "PlatMods"=w202, "Discard?"=w205) -> ()  [unwired: 1 in, 1 out]
      }
      event "SetList Table": Mouse Up {
        # "Mouse Up is now where the action happens. If up occurs over the same cell as down, it is a \"click\" and left click is called after sorting buttions.\nHowever if up occurs over a different cell than down, we do nothing and let LabVIEW give click-and-drag selection for FREE! Of course, we still\nneed to coerce selection to be within data bounds."
        n104 = event-data() -> ("CtlRef"=w224:refnum<vi>)  [unwired: 1 in, 4 out]
        n105 = call "CoerceSelection.vi"("error in (no error)"=w225, "SetList Table ref"=w224) -> ()  [unwired: 9 in, 1 out]
      }
      event "SetList Table": Shortcut Menu Activation? {
        # "No need for DeferPanUpdts here..."
        # "click within selection?"
        # "row type set after determining click is in a \nvalid column. (Mouse down? event)"
        # "Removed all right-clicks that aren't in a data column\nin Mouse Down? event..."
        n106 = event-data() -> ("CtlRef"=w247:refnum<vi>, "Coords"=w246:T13, "MenuRef"=w235:refnum<k9>)  [unwired: 1 in]
        n107 = invoke class="Tbl (strict)" method="Point To Row Column"(reference=w247, error in=w248, "Point"=w246) -> (reference out=w239:refnum<vi>, error out=w237:errorcluster, "CellPosition"=w226:T5)  [unwired: 3 in, 3 out]
        n108 = Unbundle By Name(w226) -> ("Column"=w244:i32)
        n109 = local read "Col array"() -> (w228:refnum<class "Column.lvclass">[])
        n110 = property class="Tbl (strict)"(reference=w239, error in=w237) -> (reference out=w238:refnum<vi>, error out=w236:errorcluster, "Selection Size"=w234:T5, "Selection Start"=w233:T5)
        n111 = Index Array(array=w228, index=w244) -> (element=w245:refnum<class "Column.lvclass">)
        n112 = Add(x=w234, y=w233) -> (x+y=w242:T5)
        n113 = control-ref of="Clipboard"() -> (w229:refnum<vi>)
        n114 = local read "Button\n(Mouse Down?)"() -> (w227:u16)
        n115 = Greater?(x=w242, y=w226) -> (0:w241:cluster{"Row":bool, "Column":bool})
        n116 = Less Or Equal?(x=w233, y=w226) -> (x <= y?=w240:cluster{"Row":bool, "Column":bool})
        n117 = And(x=w241, y=w240) -> (x .and. y?=w232:cluster{"Row":bool, "Column":bool})
        n118 = Cluster To Array(cluster=w232) -> (array=w231:bool[])
        n119 = And Array Elements(Boolean array=w231) -> (logical AND=w230:bool)
        "withinSelection?" <- w230
        n120 = call-dynamic "MenuBuild.vi"("Column in"=w245, "row type"="row type", "Clipboard"=w229, "MenuRef In"=w235, "Click Position"=w226, "Table CtlRef In"=w238, "error in (no error)"=w236, "withinSelection?"=w230, "Button\n(Mouse Down?)"=w227) -> ("error out"=w249:errorcluster)  [unwired: 3 in, 3 out]
        n121 = event-data() -> ()  [unwired: 2 in, 1 out]
      }
      event "SetList Table": Shortcut Menu Selection (User) {
        # "Don't check error or panel it\nmay prevent panel being updated!"
        n122 = event-data() -> ("CtlRef"=w270:refnum<vi>, "Coords"=w281:T13, "ItemTag"=w280:string)  [unwired: 1 in, 2 out]
        n123 = invoke class="Tbl (strict)" method="Point To Row Column"(reference=w270, error in=w282, "Point"=w281) -> (reference out=w252:refnum<vi>, error out=w254:errorcluster, "CellPosition"=w279:T5)  [unwired: 3 in, 3 out]
        n124 = local read "Defer Updates?"() -> (w271:bool)
        n125 = property class="Tbl (strict)"(reference=w252, error in=w254) -> (reference out=w251:refnum<vi>, error out=w253:errorcluster, "Value"=w250:string[][])
        n126 = local read "Devices queue"() -> (w257:refnum<queue>)
        n127 = call "DefPnlAndCursor.vi"("AllowDefPan? (T)"=w271, "error in (no error)"=w253, "DeferPanUpdts?"=TRUE ("DeferPanUPdts?"), "Tbl Ctrl Refnum"=w251) -> ("error out"=w258:errorcluster)  [unwired: 7 in]
        n128 = local read "DevNums"() -> (w260:i32[])
        n129 = call "ModeFromDevices.vi"("error in (no error)"=w258, "Devices queue"=w257) -> ("error out"=w259:errorcluster, "Mode Col"=w269:i32)  [unwired: 8 in]
        n130 = call "SetList SWI to Devices.vi"("error in (no error)"=w259, "SWI table"=w250, "DevNums In"=w260, "Devices queue"=w257) -> ("error out"=w255:errorcluster, "Devices queue out"=w256:refnum<queue>)  [unwired: 5 in, 1 out]
        n131 = control-ref of="VariableManager"() -> (w263:refnum<vi>)
        n132 = Unbundle By Name(w279) -> ("Column"=w276:i32)
        n133 = local read "Col array"() -> (w278:refnum<class "Column.lvclass">[])
        n134 = control-ref of="Table History"() -> (w262:refnum<vi>)
        n135 = control-ref of="Clipboard"() -> (w266:refnum<vi>)
        n136 = control-ref of="Col array"() -> (w264:refnum<vi>)
        n137 = control-ref of="Select Layout"() -> (w265:refnum<vi>)
        n138 = Index Array(array=w278, index=w276) -> (element=w277:refnum<class "Column.lvclass">)
        n139 = Bundle By Name(cluster=T14 {"Clipboard"=refnum, "Layout Ring Refnum"=refnum, "Col Array Ref in"=refnum, "VariableManagerRef"=refnum, "Table CtlRef In"=refnum, "Table History ref"=refnum, "Devices queue"=refnum} ("SetList Refs"), "Devices queue"=w256, "Clipboard"=w266, "Layout Ring Refnum"=w265, "Col Array Ref in"=w264, "VariableManagerRef"=w263, "Table CtlRef In"=w252, "Table History ref"=w262) -> (w261:T14)
        n140 = call-dynamic "MenuDo.vi"("ModeCol Index"=w269, "Cell Position"=w279, "error in (no error)"=w255, "SetList Refs"=w261, "ItemTag"=w280, "Column in"=w277) -> ("error out"=w275:errorcluster, "Update HWI?"=w268:bool)  [unwired: 1 in, 3 out]
        n141 = case shown="True" w268 {
          frame False {
          }
          frame True {
            n142 = property on="UpdateHWI Button" class="Bool (strict)"("DisabledEnum"=T11."Enabled" ("Disabled")) -> ()  [unwired: 2 in, 2 out]
          }
        }
        n143 = call "DefPnlAndCursor.vi"("AllowDefPan? (T)"=w271, "error in (no error)"=w275, "DeferPanUpdts?"=FALSE ("DeferPanUPdts?"), "Tbl Ctrl Refnum"=w252) -> ("error out"=w274:errorcluster)  [unwired: 7 in]
      }
      event "SetList Table": Mouse Enter {
        # "Change to hand inside table"
        n144 = event-data() -> ()  [unwired: 1 in, 1 out]
        n145 = call-poly <vilib>:"Set Cursor.vi"("error in (no error)"=w285, "icon"=6) -> ("error out"=w284:errorcluster)  [unwired: 8 in, 1 out]
      }
      event "SetList Table": Mouse Leave {
        # "Change back to default pointer outside table control"
        n146 = event-data() -> ()  [unwired: 1 in, 1 out]
        n147 = call-poly <vilib>:"Set Cursor.vi"("error in (no error)"=w288, "icon"=0) -> ("error out"=w287:errorcluster)  [unwired: 8 in, 1 out]
      }
      event "User defined functions": Value Change {
        # "Closing allows a user to delete\na \"defined function\" simply by \nremoving it. Then only what remains\nis re-registered.\n\n(This also throws away cached variables!)"
        n148 = event-data() -> ("OldVal"=w295:string, "NewVal"=w294:string)  [unwired: 1 in, 1 out]
        n149 = call "Caching_Expression_Evaluator_Table.vi"("method"=t_Caching_Expression_Evaluator_Methods_Table."close", "error in (no error)"=w292) -> ("error out"=w291:errorcluster)  [unwired: 11 in, 2 out]
        n150 = call "Caching_Expression_Evaluator_Table.vi"("method"=t_Caching_Expression_Evaluator_Methods_Table."execute", "expression/scriptlet"=w294, "error in (no error)"=w291) -> ("error out"=w297:errorcluster)  [unwired: 10 in, 2 out]
        n151 = case shown="No Error" w297 {
          selector: w297 -> [_ w299]
          tunnel: [_ errorcluster {"status"=FALSE, "code"=0, "source"=""} ("error out")] -> w296
          tunnel: w295 -> [_ w303]
          frame No Error {
            # "successful function \"registration\"; all other \"caching eval table\" calls will know functions now"
            n152 = property on="UpdateHWI Button" class="Bool (strict)"("DisabledEnum"=T11."Enabled" ("Disabled")) -> ()  [unwired: 2 in, 2 out]
          }
          frame Error {
            # "reset old, valid functions"
            # "on parsing error: reset functions to last, Clear error (and present warning dialog)"
            n153 = call "Caching_Expression_Evaluator_Table.vi"("method"=t_Caching_Expression_Evaluator_Methods_Table."execute", "expression/scriptlet"=w303) -> ("error out"=w301:errorcluster)  [unwired: 11 in, 2 out]
            n154 = Merge Errors(w301, w299) -> (w300:errorcluster)
            n155 = local write "User defined functions"(w303) -> ()
            n156 = disable-structure shown="Enabled" {
              disable-tunnel: w300 -> [w308 _]
              frame Enabled {
                w310 = T19 1 items=["no dialog", "OK message", "continue or stop message", "OK message + warnings", "continue/stop + warnings"] ("type of dialog (OK msg:1)")
                n157 = Unbundle By Name(w308) -> ("source"=w306:string)
                n158 = Concatenate Strings("\n*User Functions* error: \n" ("string"), w306) -> (w307:string)
                n159 = Bundle By Name(cluster=w308, "source"=w307) -> (w309:errorcluster)
                n160 = call <vilib>:"Simple Error Handler.vi"("type of dialog (OK msg:1)"=w310, "error in (no error)"=w309) -> ()  [unwired: 3 in, 5 out]
              }
              frame Disabled {
              }
            }
          }
        }
      }
      event "Select Layout": Value Change {
        n161 = event-data() -> ("NewVal"=w316:i32)  [unwired: 1 in, 2 out]
        n162 = local read "Defer Updates?"() -> (w314:bool)
        n163 = local read "Col array"() -> (w315:refnum<class "Column.lvclass">[])
        n164 = call "ApplySelectedLayout.vi"("Defer Updates? (T)"=w314, "error in (no error)"=w313, "Layout index"=w316, "Col array"=w315, "Tbl Refnum"=w311) -> ("error out"=w312:errorcluster)  [unwired: 6 in]
      }
      event "ConfigLayoutsButton": Value Change {
        # "Make sure col array is updated \nwith \"filmstrip\" sequence!"
        # "Want preview of layouts as we make them\n-->VI gets panel reference from table control to defer updates as required."
        n165 = event-data() -> ()  [unwired: 1 in, 3 out]
        n166 = disable-structure shown="Enabled" {
          frame Enabled {
            # "reset button"
            n167 = local write "ConfigLayoutsButton"(FALSE) -> ()
          }
          frame Disabled {
          }
        }
        n168 = flat-sequence {
          tunnel: w320 -> [w333]
          tunnel: [w328] -> w319
          tunnel: [w323] -> w317
          tunnel: [w337] -> w318
          tunnel: w319 -> [w338]
          tunnel: w317 -> [w334]
          frame #0 {
            n169 = local read "Devices queue"() -> (w326:refnum<queue>)
            n170 = local read "Defer Updates?"() -> (w330:bool)
            n171 = local read "DevNums"() -> (w327:i32[])
            n172 = control-ref of="Col array"() -> (w329:refnum<vi>)
            n173 = control-ref of="SetList Table"() -> (w332:refnum<vi>)
            n174 = control-ref of="Select Layout"() -> (w331:refnum<vi>)
            n175 = Dequeue Element(queue=w326) -> (queue out=w325:refnum<queue>, element=w322:refnum<class "Device.lvclass">[], error out=w324:errorcluster)  [unwired: 2 in, 1 out]
            n176 = call "GetNameList.vi"("Devices"=w322) -> ("Names in use"=w321:string[])  [unwired: 8 in, 2 out]
            n177 = Enqueue Element(queue=w325, element=w322, error in (no error)=w324) -> (queue out=w323:refnum<queue>)  [unwired: 1 in, 2 out]
            n178 = call "ConfigLayouts.vi"("DevNums"=w327, "Dev Names"=w321, "Defer Updates? (True)"=w330, "Tbl Refnum"=w332, "error in (no error)"=w333, "Col Array Refnum"=w329, "Layout Ring Refnum"=w331) -> ("error out"=w328:errorcluster)  [unwired: 4 in]
          }
          frame #1 {
            # "Need to push appearance changes\nto the columns! (or change layout\nto act on devices...)"
            n179 = local read "Col array"() -> (w336:refnum<class "Column.lvclass">[])
            n180 = local read "DevNums"() -> (w335:i32[])
            n181 = call "SetList Columns to Devices.vi"("error in (no error)"=w338, "Col array in"=w336, "DevNums In"=w335, "Devices queue"=w334) -> ("error out"=w337:errorcluster)  [unwired: 6 in, 1 out]
          }
        }
      }
      event "FitCol2Text Button": Value Change {
        # "Resizes all displayed columns"
        n182 = event-data() -> ()  [unwired: 1 in, 3 out]
        n183 = local read "Select Layout"() -> (w342:i32)
        n184 = local write "FitCol2Text Button"(FALSE ("FitCol2Text Button")) -> ()
        n185 = local read "Col array"() -> (w343:refnum<class "Column.lvclass">[])
        n186 = local read "Defer Updates?"() -> (w341:bool)
        n187 = call "FitCol2Text.vi"("Defer Updates?"=w341, "error in (no error)"=w345, "SetList Table ref"=w344, "Col array"=w343, "Select Layout"=w342) -> ("error out"=w340:errorcluster)  [unwired: 6 in]
      }
      event Value Change {
        # "Add Device is also used in Manage Devices.vi, so it was simpler\nto leave it expecting the [Devices] and dequeue-enqueue around it."
        # "Note: DevNums are used in \"Device Change to SetList.vi\""
        # "Converted to subVI so Manage can use same code for Add!"
        n188 = event-data() -> ("CtlRef"=w373:refnum<vi>)  [unwired: 1 in, 2 out]
        n189 = local read "Defer Updates?"() -> (w355:bool)
        n190 = call "DefPnlAndCursor.vi"("AllowDefPan? (T)"=w355, "error in (no error)"=w356, "DeferPanUpdts?"=TRUE ("DeferPanUPdts?"), "Tbl Ctrl Refnum"=w354) -> ("error out"=w357:errorcluster)  [unwired: 7 in]
        n191 = control-ref of="SetList Table"() -> (w366:refnum<vi>)
        n192 = property class="Tbl (strict)"(reference=w366, error in=w357) -> (reference out=w361:refnum<vi>, error out=w365:errorcluster, "Value"=w364:string[][])
        n193 = local read "Devices queue"() -> (w363:refnum<queue>)
        n194 = local read "DevNums"() -> (w362:i32[])
        n195 = local read "Col array"() -> (w372:refnum<class "Column.lvclass">[])
        n196 = control-ref of="Table History"() -> (w367:refnum<vi>)
        n197 = call "SetList SWI to Devices.vi"("error in (no error)"=w365, "SWI table"=w364, "DevNums In"=w362, "Devices queue"=w363) -> ("error out"=w349:errorcluster, "Devices queue out"=w353:refnum<queue>)  [unwired: 5 in, 1 out]
        n198 = Dequeue Element(queue=w353) -> (queue out=w351:refnum<queue>, element=w352:refnum<class "Device.lvclass">[], error out=w348:errorcluster)  [unwired: 2 in, 1 out]
        n199 = control-ref of="Select Layout"() -> (w369:refnum<vi>)
        n200 = call "AddDevice.vi"("Device List in"=w352, "Table Ref In"=w361, "Table History ref"=w367, "Layout Ref"=w369, "DevNums In"=w362, "Col array in"=w372, "error in (no error)"=w349, "Add Device"=w373) -> ("Device List out"=w350:refnum<class "Device.lvclass">[], "DevNums Out"=w370:i32[], "Col array out"=w371:refnum<class "Column.lvclass">[], "Changes Made?"=w368:bool, "error out"=w347:errorcluster)  [unwired: 3 in]
        n201 = Enqueue Element(queue=w351, element=w350, error in (no error)=w348) -> ()  [unwired: 1 in, 3 out]
        n202 = local write "DevNums"(w370) -> ()
        n203 = local write "Col array"(w371) -> ()
        n204 = call "DefPnlAndCursor.vi"("AllowDefPan? (T)"=w355, "error in (no error)"=w347, "DeferPanUpdts?"=FALSE ("DeferPanUPdts?"), "Tbl Ctrl Refnum"=w354) -> ("error out"=w359:errorcluster)  [unwired: 7 in]
        n205 = case shown="True" w368 {
          frame False {
          }
          frame True {
            n206 = property on="UpdateHWI Button" class="Bool (strict)"("DisabledEnum"=T11."Enabled" ("Disabled")) -> ()  [unwired: 2 in, 2 out]
          }
        }
      }
      event "ManageDevicesButton": Value Change {
        # "push SWI to devices (so they can operate\non it easily if column #s change)"
        n207 = event-data() -> ()  [unwired: 1 in, 3 out]
        n208 = control-ref of="SetList Table"() -> (w383:refnum<vi>)
        n209 = property class="Tbl (strict)"(reference=w383) -> (reference out=w382:refnum<vi>, error out=w380:errorcluster, "Value"=w379:string[][])  [unwired: 1 in]
        n210 = local read "Devices queue"() -> (w378:refnum<queue>)
        n211 = local read "DevNums"() -> (w381:i32[])
        n212 = call "SetList SWI to Devices.vi"("error in (no error)"=w380, "SWI table"=w379, "DevNums In"=w381, "Devices queue"=w378) -> ("Devices queue out"=w375:refnum<queue>)  [unwired: 5 in, 2 out]
        n213 = local read "DevNums"() -> (w388:i32[])
        n214 = local read "Col array"() -> (w387:refnum<class "Column.lvclass">[])
        n215 = control-ref of="Table History"() -> (w376:refnum<vi>)
        n216 = local write "ManageDevicesButton"(FALSE) -> ()
        n217 = control-ref of="Select Layout"() -> (w384:refnum<vi>)
        n218 = call "Manage Devices.vi"("Devices queue"=w375, "Table Ref In"=w382, "DevNums In"=w388, "Col array in"=w387, "Table History ref"=w376, "Layout ref"=w384) -> ("Changes Made?"=w377:bool, "DevNums Out"=w385:i32[], "Col array out"=w386:refnum<class "Column.lvclass">[])  [unwired: 1 in, 1 out]
        n219 = local write "DevNums"(w385) -> ()
        n220 = local write "Col array"(w386) -> ()
        n221 = case shown="True" w377 {
          frame False {
          }
          frame True {
            n222 = property on="UpdateHWI Button" class="Bool (strict)"("DisabledEnum"=T11."Enabled" ("Disabled")) -> ()  [unwired: 2 in, 2 out]
          }
        }
      }
      event "quit": Value Change {
        # "Need to close viewer?"
        # "store devices state on Quit.\nThis should be the ONLY local variable call!!!"
        # "Save SWI to device array. If VI is restarted, the table will be re-initialized\nfrom device array, erasing any bug-causing user edits to table control\nthe user made while VI was stopped."
        # "Stop VMUI when stopping SetList (otherwise Actor stays in memory until LabView closed.)"
        n223 = event-data() -> ("NewVal"=w404:bool)  [unwired: 1 in, 1 out]
        n224 = control-ref of="VariableManager"() -> (w396:refnum<vi>)
        n225 = control-ref of="SetList Table"() -> (w403:refnum<vi>)
        n226 = property class="Tbl (strict)"(reference=w403, error in=w398) -> (error out=w401:errorcluster, "Value"=w400:string[][])  [unwired: 1 out]
        n227 = local read "Devices queue"() -> (w399:refnum<queue>)
        n228 = local read "DevNums"() -> (w402:i32[])
        n229 = call "VMUIStop.vi"("VariableManagerRef in"=w396) -> ()  [unwired: 9 in, 2 out]
        n230 = disable-structure shown="Enabled" {
          frame Enabled {
            # "this goes a long way towards solving bug where\nvariables/functions persist after VI is stopped.\nWe'll also need to add this to Save/Load AND \nmake sure to \"nil\" deleted variables from VM."
            # "test closing Lua state"
            n231 = call "Caching_Expression_Evaluator_Table.vi"("method"=t_Caching_Expression_Evaluator_Methods_Table."close") -> ()  [unwired: 12 in, 3 out]
          }
          frame Disabled {
          }
        }
        n232 = call "SetList SWI to Devices.vi"("error in (no error)"=w401, "SWI table"=w400, "DevNums In"=w402, "Devices queue"=w399) -> ("error out"=w391:errorcluster, "Devices queue out"=w395:refnum<queue>)  [unwired: 5 in, 1 out]
        n233 = Dequeue Element(queue=w395) -> (queue out=w394:refnum<queue>, element=w392:refnum<class "Device.lvclass">[], error out=w393:errorcluster)  [unwired: 2 in, 1 out]
        n234 = local write "Devices"(w392) -> ()
        n235 = Release Queue(queue=w394, error in (no error)=w393) -> ()  [unwired: 1 in, 3 out]
        n236 = local write "quit"(FALSE ("quit")) -> ()
      }
      event "Undo": Value Change {
        n237 = event-data() -> ()  [unwired: 1 in, 3 out]
        n238 = local read "Defer Updates?"() -> (w411:bool)
        n239 = disable-structure shown="Enabled" {
          disable-tunnel: [w425 w427] -> w407
          disable-tunnel: w412 -> [w424 w427]
          disable-tunnel: w411 -> [w423 _]
          disable-tunnel: w410 -> [w422 _]
          frame Disabled {
            n240 = call "DefPnlAndCursor.vi"("AllowDefPan? (T)"=w423, "error in (no error)"=w424, "DeferPanUpdts?"=TRUE ("DeferPanUPdts?"), "Tbl Ctrl Refnum"=w422) -> ("error out"=w425:errorcluster)  [unwired: 7 in]
          }
          frame Enabled {
          }
        }
        n241 = local read "Devices queue"() -> (w408:refnum<queue>)
        n242 = local read "Col array"() -> (w418:refnum<class "Column.lvclass">[])
        n243 = control-ref of="Table History"() -> (w420:refnum<vi>)
        n244 = control-ref of="SetList Table"() -> (w421:refnum<vi>)
        n245 = call "ModeFromDevices.vi"("error in (no error)"=w407, "Devices queue"=w408) -> ("error out"=w406:errorcluster, "Mode Col"=w409:i32)  [unwired: 8 in]
        n246 = local write "Undo"(FALSE ("Undo")) -> ()
        n247 = control-ref of="Select Layout"() -> (w417:refnum<vi>)
        n248 = call "Un(Re)doTblChng.vi"("Undo/Redo"=enum16{"Undo", "Redo"}."Undo", "ModeCol Index"=w409, "Layout Ref"=w417, "error in (no error)"=w406, "Table CtlRef In"=w421, "Col Array in"=w418, "Table History ref"=w420) -> ("error out"=w414:errorcluster)  [unwired: 4 in]
        n249 = disable-structure shown="Enabled" {
          disable-tunnel: w414 -> [w431 w433]
          disable-tunnel: [w430 w433] -> w413
          disable-tunnel: w411 -> [w429 _]
          disable-tunnel: w410 -> [w428 _]
          frame Disabled {
            n250 = call "DefPnlAndCursor.vi"("AllowDefPan? (T)"=w429, "error in (no error)"=w431, "DeferPanUpdts?"=FALSE ("DeferPanUPdts?"), "Tbl Ctrl Refnum"=w428) -> ("error out"=w430:errorcluster)  [unwired: 7 in]
          }
          frame Enabled {
          }
        }
        n251 = property on="UpdateHWI Button" class="Bool (strict)"("DisabledEnum"=T11."Enabled" ("Disabled")) -> ()  [unwired: 2 in, 2 out]
      }
      event "Redo": Value Change {
        n252 = event-data() -> ()  [unwired: 1 in, 3 out]
        n253 = local read "Defer Updates?"() -> (w437:bool)
        n254 = disable-structure shown="Enabled" {
          disable-tunnel: w441 -> [w452 w454]
          disable-tunnel: [w451 w454] -> w440
          disable-tunnel: w437 -> [w450 _]
          disable-tunnel: w436 -> [w449 _]
          frame Disabled {
            n255 = call "DefPnlAndCursor.vi"("AllowDefPan? (T)"=w450, "error in (no error)"=w452, "DeferPanUpdts?"=TRUE ("DeferPanUPdts?"), "Tbl Ctrl Refnum"=w449) -> ("error out"=w451:errorcluster)  [unwired: 7 in]
          }
          frame Enabled {
          }
        }
        n256 = local read "Devices queue"() -> (w435:refnum<queue>)
        n257 = local read "Col array"() -> (w445:refnum<class "Column.lvclass">[])
        n258 = control-ref of="Table History"() -> (w447:refnum<vi>)
        n259 = control-ref of="SetList Table"() -> (w448:refnum<vi>)
        n260 = local write "Redo"(FALSE) -> ()
        n261 = call "ModeFromDevices.vi"("Devices queue"=w435) -> ("Mode Col"=w434:i32)  [unwired: 9 in, 1 out]
        n262 = control-ref of="Select Layout"() -> (w443:refnum<vi>)
        n263 = call "Un(Re)doTblChng.vi"("Undo/Redo"=enum16{"Undo", "Redo"}."Redo", "ModeCol Index"=w434, "Layout Ref"=w443, "error in (no error)"=w440, "Table CtlRef In"=w448, "Col Array in"=w445, "Table History ref"=w447) -> ("error out"=w438:errorcluster)  [unwired: 4 in]
        n264 = disable-structure shown="Enabled" {
          disable-tunnel: [w458 w460] -> w439
          disable-tunnel: w438 -> [w457 w460]
          disable-tunnel: w437 -> [w456 _]
          disable-tunnel: w436 -> [w455 _]
          frame Disabled {
            n265 = call "DefPnlAndCursor.vi"("AllowDefPan? (T)"=w456, "error in (no error)"=w457, "DeferPanUpdts?"=FALSE ("DeferPanUPdts?"), "Tbl Ctrl Refnum"=w455) -> ("error out"=w458:errorcluster)  [unwired: 7 in]
          }
          frame Enabled {
          }
        }
        n266 = property on="UpdateHWI Button" class="Bool (strict)"("DisabledEnum"=T11."Enabled" ("Disabled")) -> ()  [unwired: 2 in, 2 out]
      }
      event "Launch Viewer": Value Change {
        w467 = refnum<vi> refnum  # type specifier VI Refnum (for type only)
        # "When to close?\nAlso need to handle multiple button presses (they add calls\nto a queue which get called when Viewer \"Close\" is pressed.)"
        # "call and forget."
        # "Asynchronous viewer call (don't block execution in SetList)."
        n267 = event-data() -> ()  [unwired: 1 in, 6 out]
        n268 = control-ref of="VariableManager"() -> (w464:refnum<vi>)
        n269 = local write "Launch Viewer"(FALSE ("Launch Viewer")) -> ()
        n270 = control-ref of="Clipboard"() -> (w463:refnum<vi>)
        n271 = Open VI Reference(type specifier VI Refnum (for type only)=w467, vi path=path "Utils/Viewer.vi", options=128) -> (vi reference=w466:refnum<vi>, error out=w465:errorcluster)  [unwired: 3 in]
        n272 = call-by-ref "Start Asynchronous Call"(reference=w466, error in=w465, "SetList VariableManager ref"=w464, "SetList Clipboard ref"=w463) -> (reference out=→"Viewer VI ref":refnum<vi>)  [unwired: 10 in, 1 out]
      }
      event "Save to Disk": Value Change {
        n273 = event-data() -> ("NewVal"=w470:bool)  [unwired: 1 in, 2 out]
        n274 = case shown="True" w470 {
          frame False {
          }
          frame True {
            # "Also need to push SWI to devices prior to saving!\nWhat about HWI?"
            n275 = local read "Devices queue"() -> (w477:refnum<queue>)
            n276 = control-ref of="VariableManager"() -> (w473:refnum<vi>)
            n277 = local read "DevNums"() -> (w478:i32[])
            n278 = property on="SetList Table" class="Tbl (strict)"() -> (error out=w475:errorcluster, "Value"=w476:string[][])  [unwired: 2 in, 1 out]
            n279 = local write "Save to Disk"(FALSE ("Load from Disk")) -> ()
            n280 = property on="Select Layout" class="Ring (strict)"() -> ("Value"=w483:i32, "StringsAndValues[]"=w482:T16)  [unwired: 2 in, 2 out]
            n281 = local read "User defined functions"() -> (w481:string)
            n282 = call "SetList SWI to Devices.vi"("error in (no error)"=w475, "SWI table"=w476, "DevNums In"=w478, "Devices queue"=w477) -> ("error out"=w474:errorcluster, "Devices out"=w471:refnum<class "Device.lvclass">[])  [unwired: 5 in, 1 out]
            n283 = call "VMExport.vi"("VariableManagerRef in"=w473) -> ("VariableManagerExportCopy"=w472:refnum<class "VariableManager.lvclass">)  [unwired: 8 in, 2 out]
            n284 = Bundle By Name(cluster=T15 {"Version"="", "Devices"=[], "Select Layout"=0, "Layout:Strings And Values []"=[], "User defined functions"="", "VariableManager"=refnum}, "Version"="v1.0.0", "Devices"=w471, "Select Layout"=w483, "Layout:Strings And Values []"=w482, "User defined functions"=w481, "VariableManager"=w472) -> (w479:T15)
            n285 = call "Save_v5.vi"("error in"=w474, "Save Cluster"=w479) -> ("cancelled"=w486:bool, "Procedure Name"=w485:string, "Chosen Path"=w487:path)  [unwired: 6 in, 1 out]
            n286 = case shown="False" w486 {
              tunnel: w487 -> [w490 _]
              tunnel: w485 -> [w489 _]
              frame False {
                # "user saved!"
                n287 = local write "Procedure Name"(w489) -> ()
                n288 = control-ref of="Load Recent"() -> (w491:refnum<vi>)
                n289 = call "Load_HistoryUpdate.vi"("History ref"=w491, "New Path"=w490) -> ()  [unwired: 1 in]
              }
              frame True {
                # "user cancelled"
              }
            }
          }
        }
      }
      event "Load from Disk": Value Change {
        n290 = event-data() -> ("NewVal"=w492:bool)  [unwired: 1 in, 2 out]
        n291 = case shown="True" w492 {
          frame False {
          }
          frame True {
            # "ToDo: This is duplicate code! Change to function which takes control references; reuse on Load... .\nAlso need to initialize table from devices!!!"
            n292 = call "Load_v5.vi"() -> ("error out"=w493:errorcluster, "cancelled"=w498:bool, "Procedure Name"=w496:string, "Chosen Path"=w497:path, "Save Cluster"=w495:T15)  [unwired: 7 in]
            n293 = local write "Load from Disk"(FALSE ("Load from Disk")) -> ()
            n294 = case shown="False" w498 {
              tunnel: w497 -> [w515 _]
              tunnel: w496 -> [w514 _]
              tunnel: w495 -> [w507 _]
              tunnel: w493 -> [w506 _]
              tunnel: [FALSE ("Visible") _] -> w494
              frame False {
                # "user saved!"
                n295 = control-ref of="Load Recent"() -> (w516:refnum<vi>)
                n296 = control-ref of="SetList Table"() -> (w502:refnum<vi>)
                n297 = local write "Procedure Name"(w514) -> ()
                n298 = control-ref of="VariableManager"() -> (w503:refnum<vi>)
                n299 = property on="Loading Text" class="Str"("Visible"=TRUE) -> ()  [unwired: 2 in, 2 out]
                n300 = local read "Defer Updates?"() -> (w510:bool)
                n301 = local read "Devices queue"() -> (w501:refnum<queue>)
                n302 = call "Load_HistoryUpdate.vi"("History ref"=w516, "New Path"=w515) -> ()  [unwired: 1 in]
                n303 = control-ref of="Select Layout"() -> (w508:refnum<vi>)
                n304 = call "LoadedCluster_toSetList_v5.vi"("Devices queue"=w501, "Layout Ref"=w508, "Save Cluster"=w507, "Table Ref in"=w502, "VariableManagerRef"=w503, "error in (no error)"=w506, "Defer Updates? (T)"=w510) -> ("Loaded Version"=w509:string, "DevNums"=w511:i32[], "Col array"=w512:refnum<class "Column.lvclass">[], "User defined functions"=w500:string)  [unwired: 3 in, 2 out]
                n305 = disable-structure shown="Enabled" {
                  disable-tunnel: w500 -> [w517 w518]
                  frame Disabled {
                    n306 = local write "User defined functions"(w517) -> ()
                    n307 = global write "UserFunctions.vi" "User Functions"(w517) -> ()
                  }
                  frame Enabled {
                    n308 = property on="User defined functions" class="Str"("Val(Sgnl)"=w518) -> ()  [unwired: 2 in, 2 out]
                  }
                }
                n309 = local write "Loaded Version"(w509) -> ()
                n310 = property on="UpdateHWI Button" class="Bool (strict)"("DisabledEnum"=T11."Enabled" ("Disabled")) -> ()  [unwired: 2 in, 2 out]
                n311 = local write "DevNums"(w511) -> ()
                n312 = local write "Col array"(w512) -> ()
              }
              frame True {
                # "user cancelled"
              }
            }
            n313 = property on="Loading Text" class="Str"("Visible"=w494) -> ()  [unwired: 2 in, 2 out]
          }
        }
      }
      event "Load Recent": Value Change {
        # "ToDo: This is duplicate code! Change to function which takes control references; reuse on Load... .\nAlso need to initialize table from devices!!!"
        n314 = event-data() -> ("NewVal"=w527:string)  [unwired: 1 in, 2 out]
        n315 = String To Path(string=w527) -> (path=w523:path)
        n316 = call "Load_v5.vi"("Path (open dialog)"=w523) -> ("error out"=w521:errorcluster, "cancelled"=w526:bool, "Procedure Name"=w524:string, "Chosen Path"=w525:path, "Save Cluster"=w520:T15)  [unwired: 6 in]
        n317 = case shown="False" w526 {
          tunnel: w525 -> [w542 _]
          tunnel: w524 -> [w541 _]
          tunnel: w521 -> [w535 _]
          tunnel: w520 -> [w534 _]
          tunnel: [FALSE ("Visible") _] -> w519
          frame False {
            # "user loaded!"
            n318 = control-ref of="SetList Table"() -> (w530:refnum<vi>)
            n319 = control-ref of="VariableManager"() -> (w531:refnum<vi>)
            n320 = local write "Procedure Name"(w541) -> ()
            n321 = control-ref of="Load Recent"() -> (w543:refnum<vi>)
            n322 = local read "Defer Updates?"() -> (w538:bool)
            n323 = local read "Devices queue"() -> (w529:refnum<queue>)
            n324 = control-ref of="Select Layout"() -> (w537:refnum<vi>)
            n325 = call "Load_HistoryUpdate.vi"("History ref"=w543, "New Path"=w542) -> ()  [unwired: 1 in]
            n326 = call "LoadedCluster_toSetList_v5.vi"("Devices queue"=w529, "Layout Ref"=w537, "Save Cluster"=w534, "Table Ref in"=w530, "VariableManagerRef"=w531, "error in (no error)"=w535, "Defer Updates? (T)"=w538) -> ("Loaded Version"=w536:string, "DevNums"=w539:i32[], "Col array"=w540:refnum<class "Column.lvclass">[], "User defined functions"=w528:string)  [unwired: 3 in, 2 out]
            n327 = disable-structure shown="Enabled" {
              disable-tunnel: w528 -> [w544 w545]
              frame Disabled {
                n328 = local write "User defined functions"(w544) -> ()
                n329 = global write "UserFunctions.vi" "User Functions"(w544) -> ()
              }
              frame Enabled {
                n330 = property on="User defined functions" class="Str"("Val(Sgnl)"=w545) -> ()  [unwired: 2 in, 2 out]
              }
            }
            n331 = local write "Loaded Version"(w536) -> ()
            n332 = property on="Loading Text" class="Str"("Visible"=TRUE) -> ()  [unwired: 2 in, 2 out]
            n333 = local write "DevNums"(w539) -> ()
            n334 = local write "Col array"(w540) -> ()
          }
          frame True {
            # "user cancelled"
          }
        }
        n335 = property on="Loading Text" class="Str"("Visible"=w519) -> ()  [unwired: 2 in, 2 out]
        n336 = property on="UpdateHWI Button" class="Bool (strict)"("DisabledEnum"=T11."Enabled" ("Disabled")) -> ()  [unwired: 2 in, 2 out]
      }
      event "Load Old": Value Change {
        n337 = event-data() -> ("NewVal"=w547:bool)  [unwired: 1 in, 2 out]
        n338 = case shown="True" w547 {
          tunnel: [_ FALSE ("Load from Disk")] -> w546
          frame False {
          }
          frame True {
            n339 = local read "Old Procedure Path"() -> (w559:path)
            n340 = local read "Version Selection"() -> (w554:T3)
            n341 = local write "Load Old"(FALSE ("Load from Disk")) -> ()
            n342 = property on="Loading Text" class="Str"("Visible"=TRUE ("Load from Disk")) -> ()  [unwired: 2 in, 2 out]
            n343 = control-ref of="Old Procedure History"() -> (w568:refnum<vi>)
            n344 = control-ref of="VariableManager"() -> (w551:refnum<vi>)
            n345 = call "Load_HistoryUpdate.vi"("History ref"=w568, "New Path"=w559) -> ()  [unwired: 1 in]
            n346 = local read "Devices queue"() -> (w549:refnum<queue>)
            n347 = local read "Defer Updates?"() -> (w563:bool)
            n348 = control-ref of="SetList Table"() -> (w550:refnum<vi>)
            n349 = local read "Old HWGlobals Path"() -> (w557:path)
            n350 = call "convertOldSetlist_toCluster_v5.vi"("HW settings path"=w557, "Load pre 5.6 Globals?"=TRUE, "Procedure path"=w559, "Version Selection"=w554) -> ("Procedure Name"=w558:string, "Save Cluster"=w556:T15, "error out"=w555:errorcluster)  [unwired: 9 in]
            n351 = local write "Procedure Name"(w558) -> ()
            n352 = control-ref of="Select Layout"() -> (w564:refnum<vi>)
            n353 = call "LoadedCluster_toSetList_v5.vi"("Devices queue"=w549, "Layout Ref"=w564, "Save Cluster"=w556, "Table Ref in"=w550, "VariableManagerRef"=w551, "error in (no error)"=w555, "Defer Updates? (T)"=w563) -> ("Loaded Version"=w565:string, "DevNums"=w562:i32[], "Col array"=w561:refnum<class "Column.lvclass">[], "User defined functions"=w548:string)  [unwired: 3 in, 2 out]
            n354 = control-ref of="Old HWGlobals History"() -> (w567:refnum<vi>)
            n355 = disable-structure shown="Enabled" {
              disable-tunnel: w548 -> [w570 w571]
              frame Disabled {
                n356 = local write "User defined functions"(w570) -> ()
                n357 = global write "UserFunctions.vi" "User Functions"(w570) -> ()
              }
              frame Enabled {
                n358 = property on="User defined functions" class="Str"("Val(Sgnl)"=w571) -> ()  [unwired: 2 in, 2 out]
              }
            }
            n359 = local write "Loaded Version"(w565) -> ()
            n360 = local write "DevNums"(w562) -> ()
            n361 = local write "Col array"(w561) -> ()
            n362 = call "Load_HistoryUpdate.vi"("History ref"=w567, "New Path"=w557) -> ()  [unwired: 1 in]
            n363 = property on="UpdateHWI Button" class="Bool (strict)"("DisabledEnum"=T11."Enabled" ("Disabled")) -> ()  [unwired: 2 in, 2 out]
          }
        }
        n364 = property on="Loading Text" class="Str"("Visible"=w546) -> ()  [unwired: 2 in, 2 out]
      }
      event "Old Procedure History": Value Change {
        n365 = event-data() -> ("NewVal"=w572:string)  [unwired: 1 in, 2 out]
        n366 = String To Path(string=w572) -> (path=w573:path)
        n367 = local write "Old Procedure Path"(w573) -> ()
      }
      event "Old HWGlobals History": Value Change {
        n368 = event-data() -> ("NewVal"=w574:string)  [unwired: 1 in, 2 out]
        n369 = String To Path(string=w574) -> (path=w575:path)
        n370 = local write "Old HWGlobals Path"(w575) -> ()
      }
      event "Debug: apply appearance": Value Change {
        n371 = event-data() -> ()  [unwired: 1 in, 3 out]
        n372 = local read "Devices queue"() -> (w576:refnum<queue>)
        n373 = local read "Col array"() -> (w585:refnum<class "Column.lvclass">[])
        n374 = call "ModeFromDevices.vi"("error in (no error)"=w579, "Devices queue"=w576) -> ("error out"=w578:errorcluster, "Mode Col"=w577:i32)  [unwired: 8 in]
        n375 = control-ref of="SetList Table"() -> (w584:refnum<vi>)
        n376 = local read "Defer Updates?"() -> (w581:bool)
        n377 = control-ref of="Select Layout"() -> (w582:refnum<vi>)
        n378 = call "ApplyTableAppearance_benchmarking.vi"("Defer Updates? (T)"=w581, "Layout Ring Ref"=w582, "error in (no error)"=w578, "Mode Index"=w577, "Col Array in"=w585, "Table Ref in"=w584) -> ("error out"=w580:errorcluster)  [unwired: 4 in, 1 out]
        n379 = invoke on="Debug: apply appearance" class="Bool (strict)" method="Reinit To Default"(error in=w580) -> (error out=w583:errorcluster)  [unwired: 2 in, 2 out]
      }
      event "UpdateHWI Button": Value Change {
        n380 = event-data() -> ("CtlRef"=w593:refnum<vi>)  [unwired: 1 in, 3 out]
        n381 = property class="Bool (strict)"(reference=w593, "Value"=FALSE) -> ()  [unwired: 1 in, 2 out]
        n382 = local read "Update Event"() -> (w589:refnum<user-event>)
        n383 = Bundle(0, TRUE) -> (w586:cluster{i32, bool})  [unwired: 1 in]
        n384 = property on="SequenceHistory" class="Tbl (strict)"("Value"=string[][] [["", "-1", "Waiting", ""]] ("SequenceHistory")) -> (error out=w591:errorcluster)  [unwired: 2 in, 1 out]
        n385 = Generate User Event(user event=w589, event data cluster=w586, error in=w591) -> ()  [unwired: 1 in, 2 out]
      }
      event User Event {
        # "VariableManager Update Events"
        n386 = event-data() -> ("UpdateEvent"=w594:string)  [unwired: 1 in, 4 out]
        n387 = case shown="\"SequenceIndices\", \"UpdateEvent\", \"Variables\", Default" w594 {
          frame "SequenceIndices", "UpdateEvent", "Variables", Default {
            # "Re-enable UpdateHWI button if there is a change to VariableManager definition"
            n388 = property on="UpdateHWI Button" class="Bool (strict)"("DisabledEnum"=T11."Enabled" ("Disabled")) -> ()  [unwired: 2 in, 2 out]
          }
          frame "VariableGroups" {
          }
          frame "SequenceValues" {
          }
          frame "LastAcquireValues" {
          }
          frame "StopUI" {
          }
        }
      }
      event "Run Seq Button": Value Change {
        n389 = event-data() -> ("CtlRef"=w597:refnum<vi>, "NewVal"=w598:bool)  [unwired: 1 in, 1 out]
        n390 = case shown="True" w598 {
          tunnel: w597 -> [_ w601]
          tunnel: [_ w600] -> w596
          frame False {
          }
          frame True {
            n391 = control-ref of="VariableManager"() -> (w603:refnum<vi>)
            n392 = call "GetTotalSequenceSteps.vi"("VariableManagerRef in"=w603) -> ("error out"=w602:errorcluster, "TotalSequenceSteps"=w599:i32)  [unwired: 8 in, 1 out]
            n393 = case shown="No Error" w602 {
              selector: w602 -> [_ w637]
              tunnel: w601 -> [_ w639]
              tunnel: [_ w637] -> w600
              tunnel: w599 -> [w610 _]
              frame No Error {
                w605 = T11."Disabled" ("Disabled")
                n394 = for {
                  N: w610 -> [_]
                  tunnel: [w632] -> w609 mode=indexing
                  i -> [w636]
                  n395 = Number To Decimal String(number=w636) -> (decimal integer string=w635:string)  [unwired: 1 in]
                  n396 = Build Array("" ("element"), w635, "Waiting", "") -> (w632:string[])
                }
                n397 = property on="Run Button" class="Bool (strict)"("DisabledEnum"=w605) -> ()  [unwired: 2 in, 2 out]
                n398 = property on="Run Seq Button" class="Bool (strict)"("DisabledEnum"=w605) -> ()  [unwired: 2 in, 2 out]
                n399 = property on="RandomSequence" class="Bool (strict)"("DisabledEnum"=w605) -> ("Value"=w604:bool)  [unwired: 2 in, 2 out]
                n400 = property on="StopExperiment" class="Bool (strict)"("DisabledEnum"=T11."Enabled" ("Disabled")) -> ()  [unwired: 2 in, 2 out]
                n401 = case shown="True" w604 {
                  tunnel: w610 -> [_ w618]
                  tunnel: w609 -> [w615 w617]
                  tunnel: [w615 w616] -> w608
                  frame False {
                  }
                  frame True {
                    n402 = for {
                      N: w618 -> [w629]
                      shift-right: [w626] -> _
                      shift-left: w617 -> [w627]
                      tunnel: [w622] -> w616 mode=indexing
                      i -> [w630]
                      n403 = Random Number (0-1)() -> (number: 0 to 1=w619:dbl)
                      n404 = Subtract(x=w629, y=w630) -> (x-y=w628:i32)
                      n405 = Multiply(x=w628, y=w619) -> (x*y=w621:dbl)
                      n406 = Round Toward -Infinity(1:w621) -> (0:w620:dbl)
                      n407 = Delete From Array(array=w627, length=1, index (row)=w620) -> (deleted portion=w624:string[][], array with subset deleted=w626:string[][])  [unwired: 1 in]
                      n408 = Index Array(array=w624, index (row)=0) -> (element=w622:string[])  [unwired: 1 in]
                    }
                  }
                }
                n409 = local read "Seq. Event"() -> (w612:refnum<user-event>)
                n410 = Bundle("milliseconds to wait"=u32 0, FALSE) -> (w613:cluster{"milliseconds to wait":u32, bool})  [unwired: 1 in]
                n411 = property on="SequenceHistory" class="Tbl (strict)"("Value"=w608) -> (error out=w607:errorcluster)  [unwired: 2 in, 1 out]
                n412 = Generate User Event(user event=w612, event data cluster=w613, error in=w607) -> ()  [unwired: 1 in, 2 out]
              }
              frame Error {
                n413 = property class="Bool (strict)"(reference=w639, "Value"=FALSE) -> ()  [unwired: 1 in, 2 out]
              }
            }
          }
        }
      }
      event "Run Button": Value Change {
        n414 = event-data() -> ("NewVal"=w640:bool)  [unwired: 1 in, 2 out]
        n415 = case shown="True" w640 {
          frame False {
          }
          frame True {
            w641 = T11."Disabled" ("Disabled")
            n416 = local read "Seq. Event"() -> (w647:refnum<user-event>)
            n417 = property on="SequenceHistory" class="Tbl (strict)"("Value"=string[][] [["", "-1", "Waiting", ""]] ("SequenceHistory")) -> (error out=w643:errorcluster)  [unwired: 2 in, 1 out]
            n418 = Bundle("dimension size"=0, FALSE) -> (w648:cluster{"dimension size":i32, bool})  [unwired: 1 in]
            n419 = Generate User Event(user event=w647, event data cluster=w648, error in=w643) -> ()  [unwired: 1 in, 2 out]
            n420 = property on="Run Button" class="Bool (strict)"("DisabledEnum"=w641) -> ()  [unwired: 2 in, 2 out]
            n421 = property on="Run Seq Button" class="Bool (strict)"("DisabledEnum"=w641) -> ()  [unwired: 2 in, 2 out]
            n422 = property on="RandomSequence" class="Bool (strict)"("DisabledEnum"=w641) -> ()  [unwired: 2 in, 2 out]
            n423 = property on="StopExperiment" class="Bool (strict)"("DisabledEnum"=T11."Enabled" ("Disabled")) -> ()  [unwired: 2 in, 2 out]
          }
        }
      }
      event "Resume Button": Value Change {
        w657 = T11."Disabled" ("Disabled")
        n424 = event-data() -> ("CtlRef"=w651:refnum<vi>)  [unwired: 1 in, 2 out]
        n425 = property class="Bool (strict)"(reference=w651, "Value"=FALSE) -> ()  [unwired: 1 in, 2 out]
        n426 = local read "Seq. Event"() -> (w653:refnum<user-event>)
        n427 = Bundle("dimension size"=0, FALSE) -> (w652:cluster{"dimension size":i32, bool})  [unwired: 1 in]
        n428 = Generate User Event(user event=w653, event data cluster=w652) -> ()  [unwired: 2 in, 2 out]
        n429 = property on="Run Button" class="Bool (strict)"("DisabledEnum"=w657) -> ()  [unwired: 2 in, 2 out]
        n430 = property on="Run Seq Button" class="Bool (strict)"("DisabledEnum"=w657, "Value"=TRUE) -> ()  [unwired: 2 in, 2 out]
        n431 = property on="RandomSequence" class="Bool (strict)"("DisabledEnum"=w657) -> ()  [unwired: 2 in, 2 out]
        n432 = property on="StopExperiment" class="Bool (strict)"("DisabledEnum"=T11."Enabled" ("Disabled")) -> ()  [unwired: 2 in, 2 out]
      }
      event "SequenceHistory": Mouse Down? {
        # "Mulligan functionality"
        n433 = event-data() -> ("CtlRef"=w662:refnum<vi>, "Coords"=w661:T13)  [unwired: 1 in, 3 out]
        n434 = invoke class="Tbl (strict)" method="Point To Row Column"(reference=w662, "Point"=w661) -> (reference out=w659:refnum<vi>, "InBounds"=w658:bool, "CellPosition"=w660:T5)  [unwired: 4 in, 3 out]
        n435 = case shown="True" w658 {
          tunnel: w660 -> [_ w669]
          tunnel: w659 -> [_ w668]
          frame False {
          }
          frame True {
            # "If click in table"
            n436 = property class="Tbl (strict)"(reference=w668) -> (reference out=w665:refnum<vi>, "Value"=w664:string[][])  [unwired: 1 in, 1 out]
            n437 = Unbundle(w669) -> ("Row"=w663:i32)  [unwired: 1 out]
            n438 = Index Array(array=w664, index (row)=w663, index (col)=2 ("disabled index (col)")) -> (element=w666:string)
            n439 = case shown="\"Complete\", \"HW Error\"" w666 {
              tunnel: w665 -> [_ w671 w677]
              tunnel: w664 -> [_ w675 w681]
              tunnel: w663 -> [_ w674 w680]
              frame Default {
              }
              frame "Waiting" {
                n440 = Replace Array Subset(array=w675, new element="Complete", index (row)=w674, index (col)=2 ("disabled index (col)")) -> (w670:string[][])
                n441 = property class="Tbl (strict)"(reference=w671, "Value"=w670) -> ()  [unwired: 1 in, 2 out]
              }
              frame "Complete", "HW Error" {
                n442 = Replace Array Subset(array=w681, new element="Waiting", index (row)=w680, index (col)=2 ("disabled index (col)")) -> (w676:string[][])
                n443 = property class="Tbl (strict)"(reference=w677, "Value"=w676) -> ()  [unwired: 1 in, 2 out]
              }
            }
          }
        }
        n444 = event-data("Discard?"=w658) -> ()  [unwired: 4 in, 1 out]
      }
      event "Run/Sequence Error", "Update Error", "Table error": Value Change {
        n445 = event-data() -> ("NewVal"=w682:errorcluster)  [unwired: 1 in, 2 out]
        n446 = case shown="Error" w682 {
          frame No Error {
          }
          frame Error {
            # "If an error was generated in any part of the program, automatically open the Errors tab."
            n447 = property on="Tab Control" class="TabCtl (strict)"("Value"=T1."Errors" ("Tab Control")) -> ()  [unwired: 2 in, 2 out]
          }
        }
      }
    }
    "Table error" <- w44
    n448 = disable-structure shown="Enabled" {
      frame Enabled {
        # "diagnositc"
        n449 = local read "Table History"() -> (w49:T8)
        n450 = Unbundle By Name(w49) -> ("OldTable Array"=w48:T9)
        n451 = Array Size(array=w48) -> (size(s)=→"Hist. size":i32)
      }
      frame Disabled {
      }
    }
  }
  n452 = while {
    stop <- w684 stop-if-true
    # "Update Event Structure"
    n453 = local read "Dyn. Regist. Update Event"() -> (w685:refnum<event-registration>)
    n454 = event shown="[0] <Update Event>: User Event" {
      selector: w685 -> [_ _]
      dyn-events: _ -> [_ _]
      timeout: _ -> [_ _]
      tunnel: [_ w733] -> w684
      event User Event {
        n455 = event-data() -> ("Seq. Idx"=w686:i32, "Force?"=w687:bool)  [unwired: 1 in]
        n456 = case shown="True" w687 {
          tunnel: [_ w715] -> w688
          tunnel: w686 -> [_ w694]
          frame False {
          }
          frame True {
            # "prepend filenumber placeholder\n(overwritten in CycleX loop)"
            n457 = property on="SequenceHistory" class="Tbl (strict)"() -> ("Value"=w697:string[][])  [unwired: 2 in, 2 out]
            n458 = control-ref of="VariableManager"() -> (w710:refnum<vi>)
            n459 = Index Array(array=w697, index (row)=w694, index (col)=1 ("disabled index (col)")) -> (element=w698:string)
            n460 = Scan From String(format string="%d", input string=w698) -> (output 1=w693:i32)  [unwired: 3 in, 3 out]
            n461 = call "GetVariableValues.vi"("SequenceStep"=w693, "VariableManagerRef in"=w710) -> ("error out"=w707:errorcluster, "VariableValues"=w705:refnum<class "VariableValue.lvclass">[])  [unwired: 7 in, 1 out]
            n462 = control-ref of="SetList Table"() -> (w718:refnum<vi>)
            n463 = for {
              tunnel: w705 -> [w722] mode=indexing
              tunnel: [w723] -> w706 mode=indexing
              tunnel: [w721] -> w704 mode=indexing
              n464 = call "VariableValueToCluster.vi"("VariableValue"=w722) -> ("VariableValueCluster"=w721:cluster{"Name":string, "Value":dbl})  [unwired: 10 in]
              n465 = call "VariableValueToString.vi"("VariableValue"=w722) -> ("VariableValueString"=w723:string)  [unwired: 10 in]
            }
            n466 = Greater?(x=w693, y=-1) -> (0:w712:bool)
            n467 = property class="Tbl (strict)"(reference=w718, error in=w707) -> (error out=w708:errorcluster, "Value"=w714:string[][], "Column Headers[]"=w713:string[])  [unwired: 1 out]
            n468 = local read "Devices queue"() -> (w720:refnum<queue>)
            n469 = local read "DevNums"() -> (w719:i32[])
            n470 = Concatenate Strings(w706) -> (w702:string)
            n471 = call "SetList SWI to Devices.vi"("error in (no error)"=w708, "SWI table"=w714, "DevNums In"=w719, "Devices queue"=w720) -> ("error out"=w716:errorcluster, "Devices queue out"=w717:refnum<queue>)  [unwired: 5 in, 1 out]
            n472 = invoke on="SequenceHistory" class="Tbl (strict)" method="Set Cell Value"("X Index"=3 ("disabled index (col)"), "Y Index"=w694, "Value"=w702) -> ()  [unwired: 3 in, 6 out]
            n473 = call "SetList_ToString.vi"("Column Names"=w713, "Current  Variables"=w704, "Device Data"=w714) -> ("Igor Inform String"=w709:string)
            n474 = local read "Additional wait time (s)"() -> (w692:dbl)
            n475 = case shown="True" w712 {
              tunnel: w710 -> [w730 _]
              tunnel: w694 -> [w726 _]
              tunnel: w709 -> [w727 w732]
              tunnel: [w729 w731] -> w700
              frame True {
                n476 = call "Construct Sequence Variable Igor String.vi"("Current index"=w726, "VariableManagerRef"=w730) -> ("Igor Instruction String"=w728:string[])  [unwired: 9 in]
                n477 = Build Array (concatenate)(w728, w727) -> (w729:string[])
              }
              frame False {
                n478 = Build Array(w732) -> (w731:string[])
              }
            }
            n479 = call "Update HWI.vi"("Error In"=w716, "Current Variables"=w704, "Devices queue"=w717) -> ("Error Out"=w715:errorcluster, "Total Time"=w691:dbl)  [unwired: 1 in, 1 out]
            n480 = property on="Update Error" class="Clust (strict)"("Val(Sgnl)"=w715) -> ()  [unwired: 2 in, 2 out]
            n481 = case shown="..-1" w693 {
              tunnel: w715 -> [_ w724]
              frame 0, Default {
              }
              frame ..-1 {
                n482 = case shown="No Error" w724 {
                  frame No Error {
                    n483 = property on="UpdateHWI Button" class="Bool (strict)"("DisabledEnum"=T11."Disabled and Grayed Out" ("Disabled")) -> ()  [unwired: 2 in, 2 out]
                  }
                  frame Error {
                  }
                }
              }
            }
            n484 = Add(x=w691, y=w692) -> (x+y=→"Cycle Time (s)":dbl)
            n485 = Build Array (concatenate)("FileNumber=null\n", w700) -> (→"Igor Inform Array":string[])
          }
        }
        n486 = local read "Update Notifier"() -> (w689:refnum<notifier>)
        n487 = Send Notification(notification=w688, notifier=w689) -> ()  [unwired: 1 in, 2 out]
      }
      event "quit": Value Change {
        # "Tried adding local variable read of Quit outside event loop, but I think it wasn't being read properly.\nIs there a problem having three event loops checking quit? - CDH\nI think if you wanted it to work as intended with the read outside of the loop, you would need to set a timeout value and event case. - ZES"
        n488 = event-data() -> ("NewVal"=w733:bool)  [unwired: 1 in, 1 out]
      }
    }
  }
  n489 = property on="UpdateHWI Button" class="Bool (strict)"("DisabledEnum"=T11."Disabled and Grayed Out" ("Disabled")) -> ()  [unwired: 2 in, 2 out]
  n490 = property on="Loading Text" class="Str"("Visible"=FALSE ("Load from Disk")) -> ()  [unwired: 2 in, 2 out]
  n491 = case shown="False" "PreserveHist?" {
    frame False {
      w734 = T8 {"OldTable Array"=[], "Undo pointer"=0}  # Table History
      # "re-initialize to empty\nfor now"
      n492 = local write "Table History"(w734) -> ()
    }
    frame True {
    }
  }
  n493 = while {
    stop <- w735 stop-if-true
    # "Sequence Event Structure"
    n494 = local read "Dyn.\nRegist.\nSeq.\nEvent"() -> (w736:refnum<event-registration>)
    n495 = event shown="[0] <Seq Event>: User Event" {
      selector: w736 -> [_ _]
      dyn-events: _ -> [_ _]
      timeout: _ -> [_ _]
      tunnel: [_ w779] -> w735
      event User Event {
        n496 = event-data() -> ()  [unwired: 1 in, 2 out]
        n497 = property on="StopExperiment" class="Bool (strict)"() -> ("Value"=w737:bool)  [unwired: 2 in, 2 out]
        n498 = case shown="False" w737 {
          frame False {
            # "If running cycle, do not force update."
            # "Look for waiting sequence"
            # "Run Experiment"
            n499 = property on="SequenceHistory" class="Tbl (strict)"() -> ("Value"=w745:string[][])  [unwired: 2 in, 2 out]
            n500 = Index Array(array=w745, index (col)=2 ("disabled index (col)")) -> (element=w747:string[])  [unwired: 1 in]
            n501 = for {
              tunnel: w747 -> [w751] mode=indexing
              tunnel: [w749] -> w744
              tunnel: [w748] -> w742
              i -> [w748]
              stop <- w749 stop-if-true
              n502 = Equal?(x=w751, y="Waiting") -> (x = y?=w749:bool)
            }
            n503 = property on="SequenceHistory" class="Tbl (strict)"() -> ("Value"=w738:string[][])  [unwired: 2 in, 2 out]
            n504 = Index Array(array=w738, index (row)=w742, index (col)=1 ("disabled index (col)")) -> (element=w741:string)
            n505 = Not Equal?(x=w741, y="-1") -> (x != y?=w739:bool)
            n506 = case shown="True" w744 {
              tunnel: w742 -> [_ w756]
              tunnel: w739 -> [_ w755]
              frame False {
                w753 = T11."Enabled" ("Disabled")
                w754 = FALSE
                # "No waiting sequence"
                n507 = property on="Run Button" class="Bool (strict)"("Value"=w754, "DisabledEnum"=w753) -> ()  [unwired: 2 in, 2 out]
                n508 = property on="Run Seq Button" class="Bool (strict)"("Value"=w754, "DisabledEnum"=w753) -> ()  [unwired: 2 in, 2 out]
                n509 = property on="RandomSequence" class="Bool (strict)"("DisabledEnum"=w753) -> ()  [unwired: 2 in, 2 out]
                n510 = property on="StopExperiment" class="Bool (strict)"("Value"=w754, "DisabledEnum"=T11."Disabled and Grayed Out" ("Disabled")) -> ()  [unwired: 2 in, 2 out]
              }
              frame True {
                # "Run waiting  sequence"
                n511 = stacked-sequence {
                  seq-local: [_ w762 _ _] -> [_ _ _ w772]
                  tunnel: w756 -> [w758 w761 w769 w771]
                  tunnel: w755 -> [_ w760 _ _]
                  frame #0 {
                    # "Update SequenceHistory Status"
                    n512 = invoke on="SequenceHistory" class="Tbl (strict)" method="Set Cell Value"("X Index"=2 ("disabled index (col)"), "Y Index"=w758, "Value"="Programming") -> ()  [unwired: 3 in, 6 out]
                  }
                  frame #1 {
                    # "Row number of waiting sequence"
                    n513 = local read "Update Event"() -> (w767:refnum<user-event>)
                    n514 = local read "Update Notifier"() -> (w764:refnum<notifier>)
                    n515 = Bundle(w761, w760) -> (w766:cluster{i32, bool})  [unwired: 1 in]
                    n516 = Generate User Event(user event=w767, event data cluster=w766) -> (error out=w763:errorcluster)  [unwired: 2 in, 1 out]
                    n517 = Wait on Notification(notifier=w764, ignore previous (F)=TRUE, error in (no error)=w763) -> (notification=w762:errorcluster)  [unwired: 1 in, 3 out]
                  }
                  frame #2 {
                    # "Update SequenceHistory Status"
                    n518 = invoke on="SequenceHistory" class="Tbl (strict)" method="Set Cell Value"("X Index"=2 ("disabled index (col)"), "Y Index"=w769, "Value"="Executing") -> ()  [unwired: 3 in, 6 out]
                  }
                  frame #3 {
                    n519 = local read "CycleX Event"() -> (w774:refnum<user-event>)
                    n520 = Bundle(w771, FALSE) -> (w775:cluster{i32, bool})  [unwired: 1 in]
                    n521 = Generate User Event(user event=w774, event data cluster=w775, error in=w772) -> ()  [unwired: 1 in, 2 out]
                  }
                }
              }
            }
          }
          frame True {
            w777 = T11."Enabled" ("Disabled")
            w778 = FALSE
            # "Stop experiment when Stop request"
            n522 = property on="Run Button" class="Bool (strict)"("Value"=w778, "DisabledEnum"=w777) -> ()  [unwired: 2 in, 2 out]
            n523 = property on="Run Seq Button" class="Bool (strict)"("Value"=w778, "DisabledEnum"=w777) -> ()  [unwired: 2 in, 2 out]
            n524 = property on="RandomSequence" class="Bool (strict)"("DisabledEnum"=w777) -> ()  [unwired: 2 in, 2 out]
            n525 = property on="StopExperiment" class="Bool (strict)"("Value"=w778, "DisabledEnum"=T11."Disabled and Grayed Out" ("Disabled")) -> ()  [unwired: 2 in, 2 out]
          }
        }
      }
      event "quit": Value Change {
        n526 = event-data() -> ("NewVal"=w779:bool)  [unwired: 1 in, 1 out]
      }
    }
  }
  n527 = invoke on="quit" class="Bool (strict)" method="Reinit To Default"() -> ()  [unwired: 3 in, 3 out]
  n528 = while {
    i -> [w784]
    stop <- w780 stop-if-true
    # "Diagnostics..."
    n529 = flat-sequence {
      tunnel: [w793] -> w781
      frame #0 {
        n530 = Wait (ms)(milliseconds to wait=u32 100) -> ()  [unwired: 1 out]
      }
      frame #1 {
        n531 = property on="SetList Table" class="Tbl (strict)"() -> (error out=w789:errorcluster, "OwningVI"=w791:refnum<vi>)  [unwired: 2 in, 1 out]
        n532 = property on="SetList Table" class="Tbl (strict)"() -> ("Key Focus"=→"Key Focus":bool, "EditPos"=→"Edit Position":T5, "Selection Size"=→"Selection Size":T5, "Selection Start"=→"Selection Start":T5, "Index Values"=→"Index Values":T4)  [unwired: 2 in, 2 out]
        n533 = local read "quit"() -> (w793:bool)
        n534 = property class="VI"(reference=w791, error in=w789) -> (error out=w788:errorcluster, "Panel"=w790:refnum<vi>)  [unwired: 1 out]
        n535 = property class="Pnl"(reference=w790, error in=w788) -> ("DeferPanUpdts"=→"Defer Pnl Upd":bool)  [unwired: 2 out]
        n536 = local write "Val Change"(FALSE ("Val Change")) -> ()
      }
    }
    n537 = Not(x="Diag. loop?") -> (.not. x?=w782:bool)
    n538 = Or(x=w781, y=w782) -> (x .or. y?=w780:bool)
    "diag. loop cnt" <- w784
  }
  n539 = while {
    stop <- w798 stop-if-true
    # "Handles running CycleX, which runs once per step"
    n540 = local read "Dyn.\nRegist.\nCycleX\nEvent"() -> (w799:refnum<event-registration>)
    n541 = event shown="[0] <CycleX Event>: User Event" {
      selector: w799 -> [_ _]
      dyn-events: _ -> [_ _]
      timeout: _ -> [_ _]
      tunnel: [_ w843] -> w798
      event User Event {
        # "log file number"
        # "replace file number"
        n542 = event-data() -> ("Seq. Idx"=w800:i32)  [unwired: 1 in, 1 out]
        n543 = local read "File Number"() -> (w803:i32)
        n544 = Format Into String(format string="%d", w803) -> (resulting string=w801:string)  [unwired: 2 in, 1 out]
        n545 = local read "Igor Inform Array"() -> (w811:string[])
        n546 = invoke on="SequenceHistory" class="Tbl (strict)" method="Set Cell Value"("X Index"=0, "Y Index"=w800, "Value"=w801) -> ()  [unwired: 3 in, 6 out]
        n547 = Increment(x=w803) -> (x+1=w815:i32)
        n548 = local write "File Number"(w815) -> ()
        n549 = shared-variable ".\\VariableLibrary.lvlib\\FileNum"(w815) -> ()  [unwired: 1 in, 1 out]
        n550 = Concatenate Strings("FileNumber=" ("string"), w801, "\n" ("string")) -> (w805:string)
        n551 = Replace Array Subset(array=w811, new element=w805, index=0) -> (w809:string[])
        n552 = Concatenate Strings(w809) -> (w816:string)
        "Igor Inform String" <- w816
        n553 = Build Array(w816) -> (w812:string[])
        n554 = local read "Devices queue"() -> (w821:refnum<queue>)
        n555 = call "CycleX.vi"("Devices queue"=w821, "Program only changes"="Program only changes", "Program during MOT loading"="Program during MOT loading", "Igor Inform String"=w812, "Additional wait time (s)"="Additional wait time (s)") -> ("error out"=w808:errorcluster)  [unwired: 10 in]
        n556 = case shown="No Error" w808 {
          tunnel: [w830 "HW Error"] -> w817
          frame No Error {
            # "If cycle run,\nwait again"
            n557 = property on="SequenceHistory" class="Tbl (strict)"() -> ("Value"=w829:string[][])  [unwired: 2 in, 2 out]
            n558 = Index Array(array=w829, index (row)=0, index (col)=1 ("disabled index (col)")) -> (element=w828:string)
            n559 = property on="Cycle" class="Bool (strict)"() -> ("Value"=w826:bool)  [unwired: 2 in, 2 out]
            n560 = Equal?(x="-1", y=w828) -> (x = y?=w825:bool)
            n561 = And(x=w826, y=w825) -> (x .and. y?=w822:bool)
            n562 = case shown="False" w822 {
              tunnel: ["Complete" "Waiting"] -> w830
              frame False {
              }
              frame True {
              }
            }
          }
          frame Error {
            # "don't want \"complete\" if error!"
          }
        }
        n563 = invoke on="SequenceHistory" class="Tbl (strict)" method="Set Cell Value"("X Index"=2 ("disabled index (col)"), "Y Index"=w800, "Value"=w817) -> (error out=w814:errorcluster)  [unwired: 3 in, 5 out]
        n564 = case shown="Error" w808 {
          selector: w808 -> [w836 w842]
          tunnel: w814 -> [_ _]
          frame No Error {
            n565 = local read "Seq. Event"() -> (w837:refnum<user-event>)
            n566 = Bundle("milliseconds to wait"=u32 0, FALSE) -> (w838:cluster{"milliseconds to wait":u32, bool})  [unwired: 1 in]
            n567 = Generate User Event(user event=w837, event data cluster=w838, error in=w836) -> ()  [unwired: 1 in, 2 out]
          }
          frame Error {
            w840 = T11."Enabled" ("Disabled")
            w839 = FALSE
            n568 = property on="Run/Sequence Error" class="Clust (strict)"("Val(Sgnl)"=w842) -> ()  [unwired: 2 in, 2 out]
            n569 = property on="Run Button" class="Bool (strict)"("Value"=w839, "DisabledEnum"=w840) -> ()  [unwired: 2 in, 2 out]
            n570 = property on="Run Seq Button" class="Bool (strict)"("Value"=w839, "DisabledEnum"=w840) -> ()  [unwired: 2 in, 2 out]
            n571 = property on="RandomSequence" class="Bool (strict)"("DisabledEnum"=w840) -> ()  [unwired: 2 in, 2 out]
            n572 = property on="StopExperiment" class="Bool (strict)"("Value"=w839, "DisabledEnum"=T11."Disabled and Grayed Out" ("Disabled")) -> ()  [unwired: 2 in, 2 out]
          }
        }
      }
      event "quit": Value Change {
        n573 = event-data() -> ("NewVal"=w843:bool)  [unwired: 1 in, 1 out]
      }
    }
  }
